vi "TabConAlt v0.2.vi"() -> ()   [LabVIEW 2017]
uses:
  <vilib>/Platform/TimedLoop/XDataNode/timing_clust.ctl
  <vilib>/Platform/TimedLoop/XDataNode/nitl_modes.ctl
  <vilib>/Platform/TimedLoop/XDataNode/wakeup.ctl
  <vilib>/Platform/TimedLoop/scheduler/LVUserAPI/_suppVIs/Create_1kHz_TSource.vi
  <vilib>/platform/TimedLoop/XDataNode/XDataNode.xnode
  <vilib>/ErrorRing/Error Ring.xnode
  <instrlib>/Stanford Research SR865/Stanford Research SR865.lvlib
  support/LIAinteraction/LIAinteraction.lvlib
  <vilib>/Platform/TimedLoop/XDataNode/XDNodeRunTimeDep.lvlib
panel:
  out "strMAT":string="Disconnected"
  in  "initMAT":bool
  out "statusMAT":bool
  out "connMAT":bool caption="Matisse TX"
  out "strMIL":string="Disconnected"
  in  "initMIL":bool
  out "statusMIL":bool
  out "connMIL":bool caption="Millenia eV 25W"
  out "strCCD":string="Disconnected"
  in  "initCCD":bool
  out "statusCCD":bool
  out "connCCD":bool caption="Pylon CCD"
  out "strSPT":string="Disconnected"
  in  "initSPT":bool caption="Spectrometer"
  out "statusSPT":bool
  out "connSPT":bool caption="Spectrometer"
  out "strLIA":string="Disconnected"
  in  "initLIA":bool caption="Lock-in"
  out "statusLIA":bool
  out "connLIA":bool caption="Lock-in & Chopper"
  in  "initALL":bool caption="Initialize all"
  in  "stopExecution":bool
  in  "clearNotifications":bool
  out "Notifications":string="\r\r\n"
  out "measRUN":bool caption="Measurement running"
  out "measREADY":bool caption="Measurement ready"
  out "UIbusy":bool caption="Interface busy"
  in  "Settings":T1(tab)=enum."Interface"
  in  "visaSPT":string caption="VISA address"
  in  "visaCCD":string caption="VISA address"
  out "unitChopFreq":string="Hz"
  in  "Linear ramp":dbl[unit]=200.0 min=1.0 max=500.0 step=1.0 format="%#_4g"
  in  "Start chopping":bool
  in  "findPrime":bool
  in  "visaLIA":string="visa://10.132.193.16/GPIB0::28::INSTR" caption="VISA address"
  in  "Chopping Frequency":dbl(knob)=1037.3807522912232 min=200.0 max=2000.0 step=1.0 scale=200.0..2000.0
  out "unitLinearRamp":string="Hz/s"
  in  "Ring cavity  energy":cluster{dbl[unit], dbl[unit]}(slide) caption="Ring cavity  energy / eV"
  in  "Ring cavity wavelength":cluster{dbl[unit], dbl[unit]}(slide)={0.0, 9.616279069767442e-07} caption="Ring cavity wavelength / nm"
  in  "Enslave Millennia eV":bool
  in  "Installed Optics":string(combo)="MOS2 BB"
  in  "visaMAT":string caption="VISA address"
  in  "Matisse Power":dbl[unit](knob)=1e-06 caption="Millenia Power" min=1.0 max=25.0 scale=1.0..25.0
  in  "visaMIL":string caption="VISA address"
  in  "Millenia Power":dbl[unit](knob)=0.001 min=1.0 max=25.0 scale=1.0..25.0
  in  "Hidden indicators":enum32{"General", "Sync"}(tab)
  out "LIAtimer1":bool
  out "TestInd2":bool
  out "MeasNum":dbl
  out "instrNum":dbl
  in  "actDummy":bool=TRUE
  out "DummyVisaOut":string
  in  "mainqSize":dbl=1000.0 caption="Queue size" min=1.0 step=1.0
  in  "timebaseMaster":dbl[unit]=0.08 caption="Master timebase" min=0.0001 max=0.5 step=0.0001 format="%#_6f"
  in  "timebaseSlave":dbl[unit]=0.16 caption="Slave timebase" min=0.0001 max=0.5 step=0.0001
  in  "abbrSPT":string="SPT"
  in  "abbrCCD":string="CCD"
  in  "abbrMIL":string="MIL"
  in  "abbrMAT":string="MAT"
  in  "abbrLIA":string="LIA"
  in  "nameSPT":string="Spectrometer"
  in  "nameLIA":string="SRS865"
  in  "nameCCD":string="Pylon CCD"
  in  "nameMIL":string="Millennia eV 25W"
  in  "nameMAT":string="Matisse 2 TX"
  # "Lower"
  # "Upper"
  # "eV"
  # "eV"
  # "Lower"
  # "Upper"
  # "nm"
  # "nm"
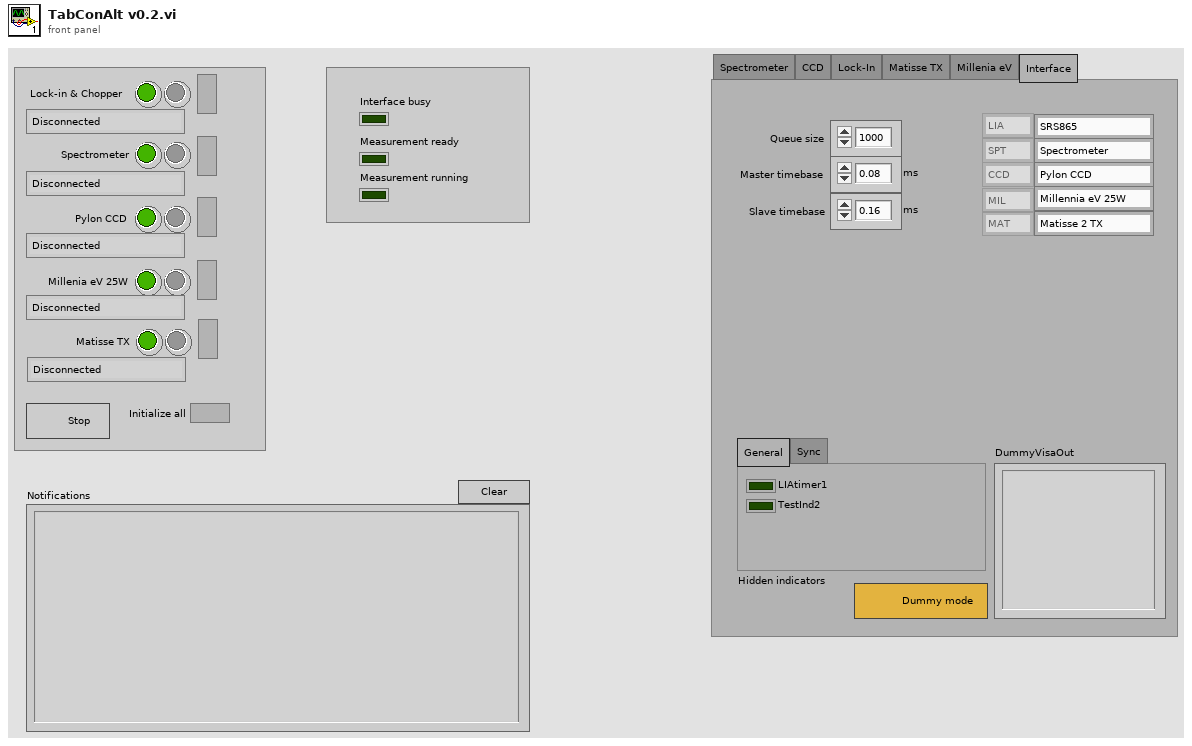
[diagram p1: front panel]
types:
  T1 = enum32{"Spectrometer", "CCD", "Lock-In", "Matisse TX", "Millenia eV", "Interface"}
  T2 = cluster{"elementArr":cluster{"cmd":string, "cmdclass":string, "data":variant}[]}
  T3 = cluster{"str":string, "ctlref":refnum<vi>, "newStatus":bool, "ctlstr":refnum<vi>}
  T4 = cluster{string, "chgStatusLED":refnum<user-event>}
  T5 = cluster{cluster{string, "chgStatusLED":refnum<user-event>}, cluster{string, "qintoMain":refnum<user-event>}}
  T6 = typedef "XDNodeRunTimeDep.lvlib/timing_clust.ctl" = cluster{"Expected End [f-1]":u64, "Actual End [f-1]":u64, "Finished Late? [f-1]":bool, "Expected End [i-1]":u64, "Actual End [i-1]":u64, "Finished Late? [i-1]":bool, "Expected Start [i]":u64, "Actual Start [i]":u64, "Expected Start [f]":u64, "Actual Start [f]":u64, "Source Name":string, "Structure Name":string, "Period":i64, "Deadline":i64, "Offset":i64, "Start":i64, "Priority":i32, "Timeout":i32, "Mode":T7, "Wakeup Reason":T8, "Error":errorcluster, "Source Type":string, "Secondary Source Type":string, "Global End Time":u64, "Global Start Time":u64, "Frame Duration":u64, "Iteration Duration":u64, "Assigned CPU":i32, "I/O Scan Engine Mode":u32}
  T7 = typedef "XDNodeRunTimeDep.lvlib/nitl_modes.ctl" = enum32{"No Change", "Process missed periods, maintain original phase", "Discard missed periods, maintain original phase", "Process missed periods, ignore original phase", "Discard missed periods, ignore original phase"}
  T8 = typedef "XDNodeRunTimeDep.lvlib/wakeup.ctl" = enum32{"Normal", "Aborted", "Asynchronous wakeup", "Timing source error", "Timed loop error", "Timeout"}
  T9 = typedef "RefArray.ctl" = cluster{"String":string, "Array":refnum<vi>[]}[]
  T10 = cluster{"Command":string, "Command class":string, "Variant":variant}
  T11 = cluster{"Command":string, "Command class":string, "Variant":variant}[]
  T12 = cluster{"cmd":string, "cmdclass":string, "data":variant}[]
  T13 = typedef "eventsource.ctl" = u32
  T14 = cluster{string, "abbrMAT":string, "Variant":variant}
  T15 = cluster{string, "abbrMAT":string, "Variant":variant}[]
  T16 = cluster{"String":string, "String 2":string, "Variant":variant}[]
  T17 = cluster{"String":string, "_chgStatusLED":refnum<user-event>}
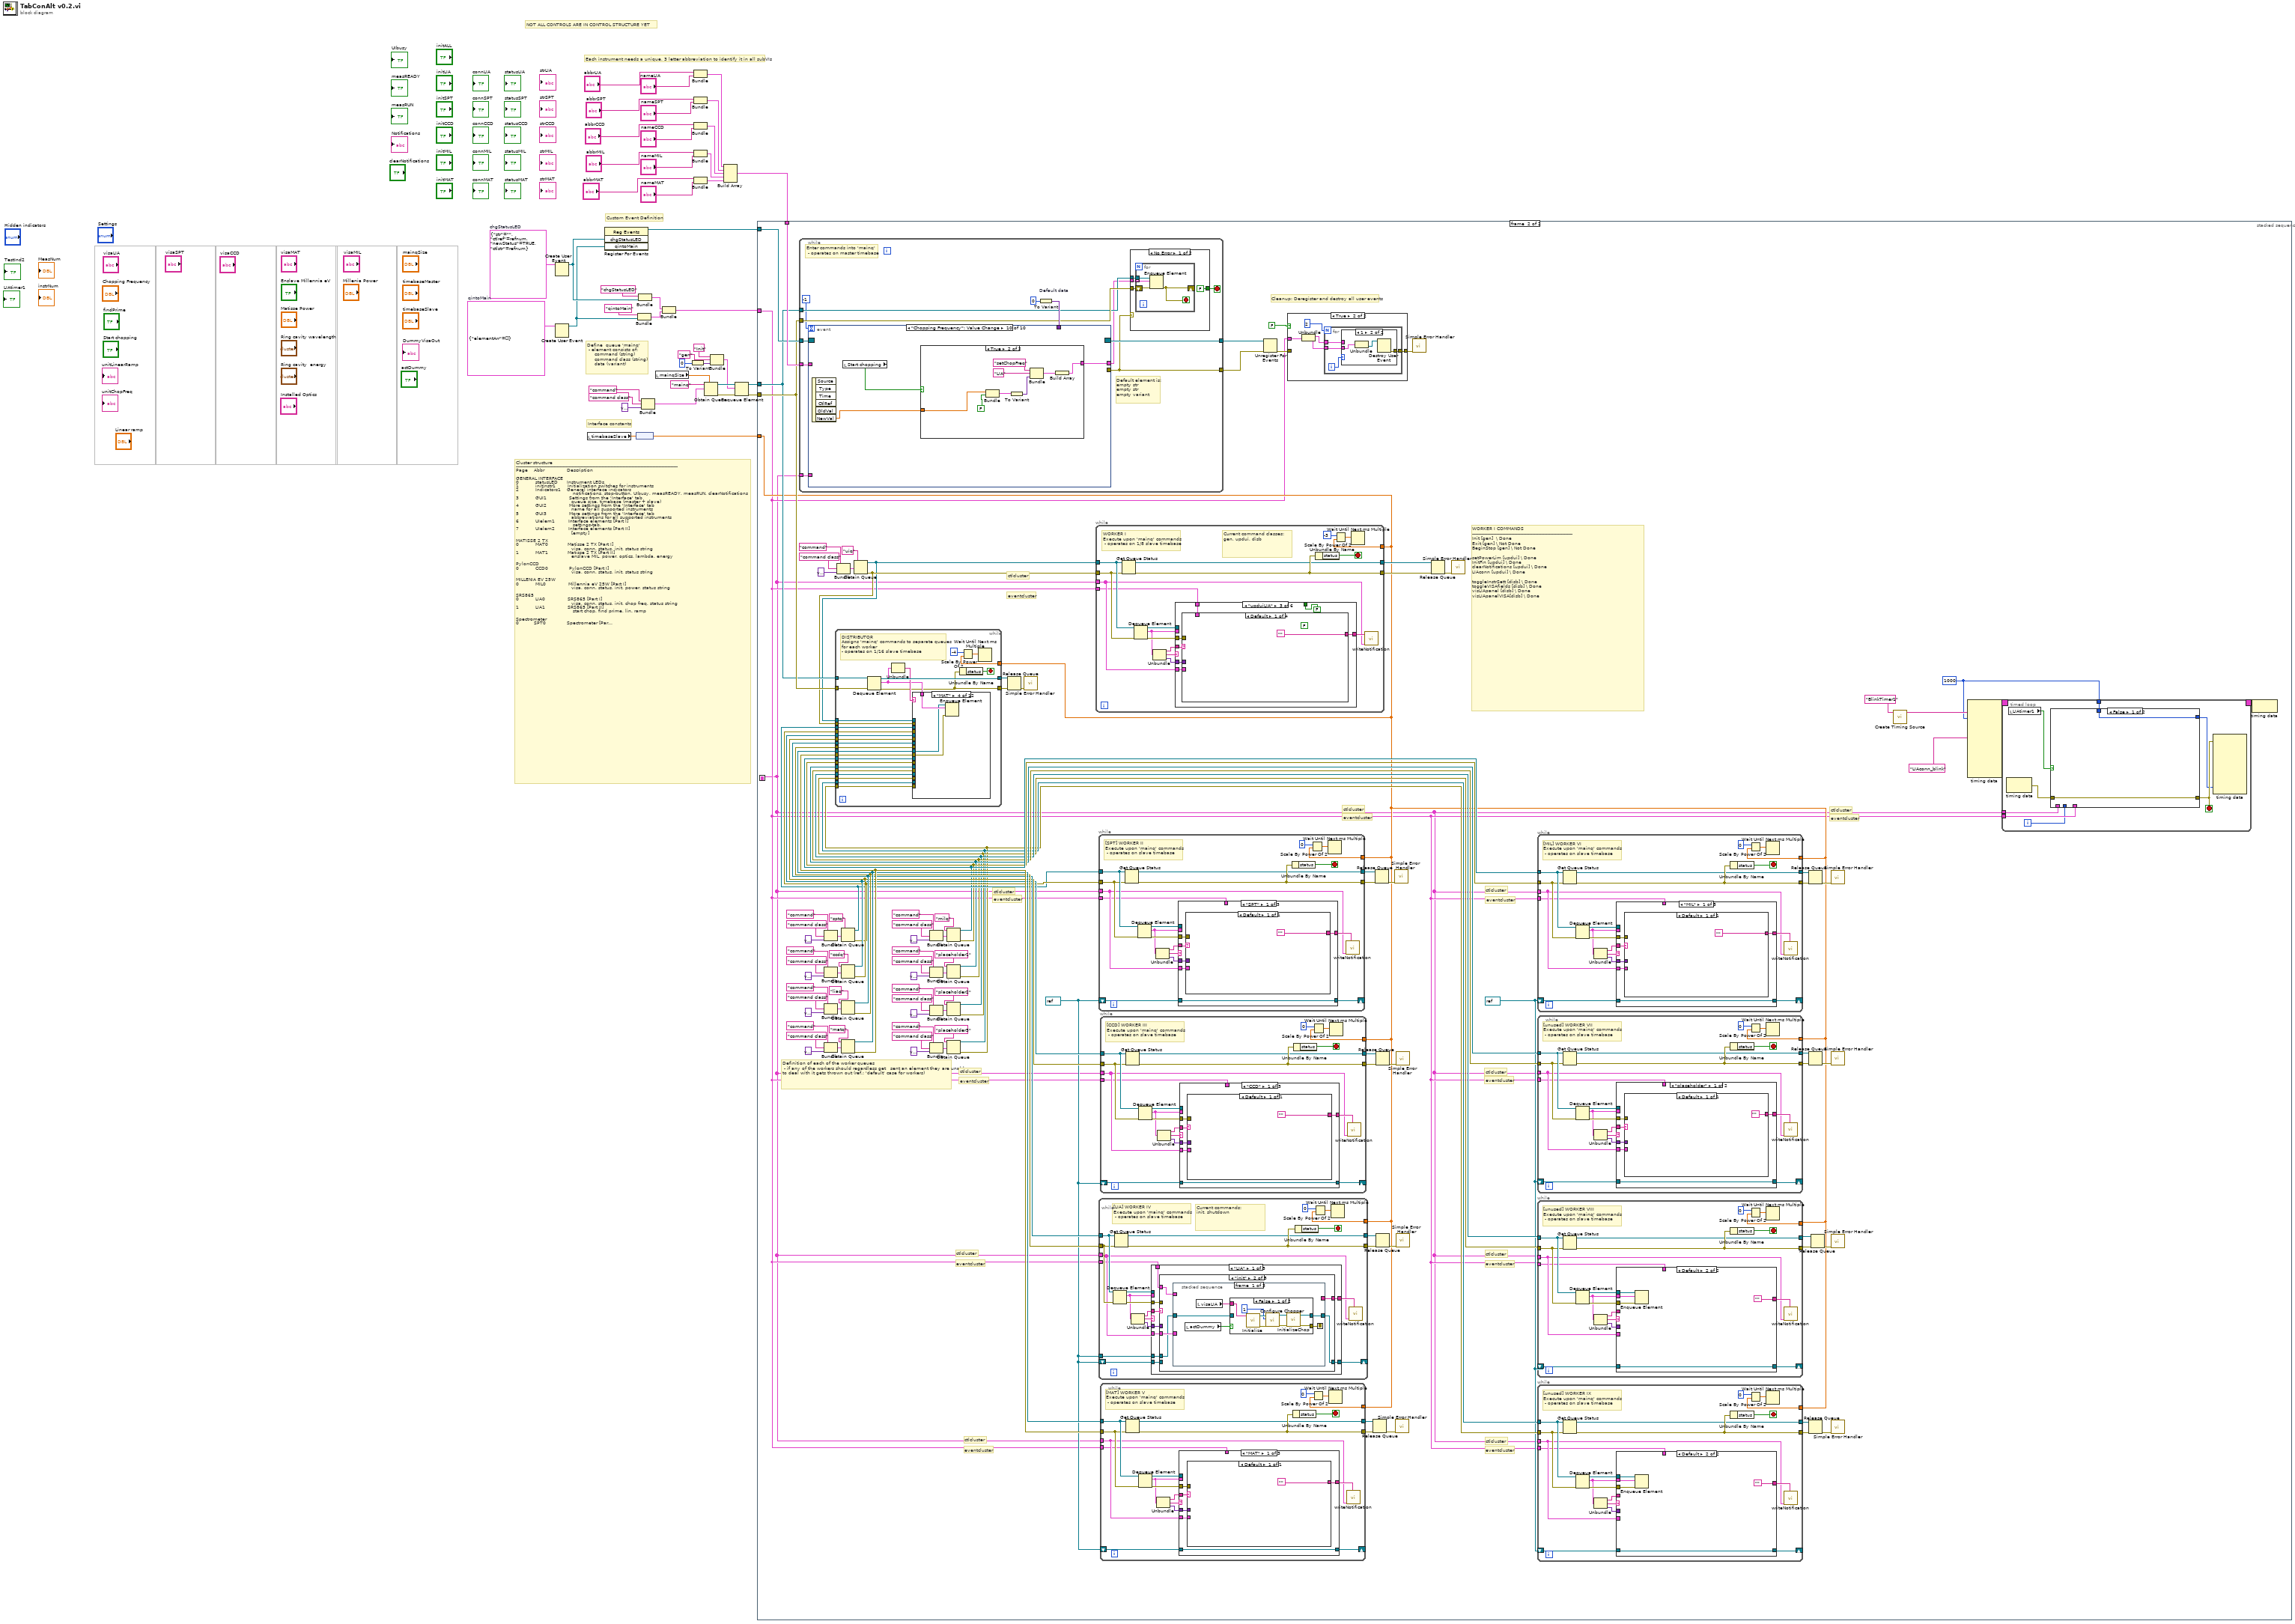
[diagram p0: block diagram]
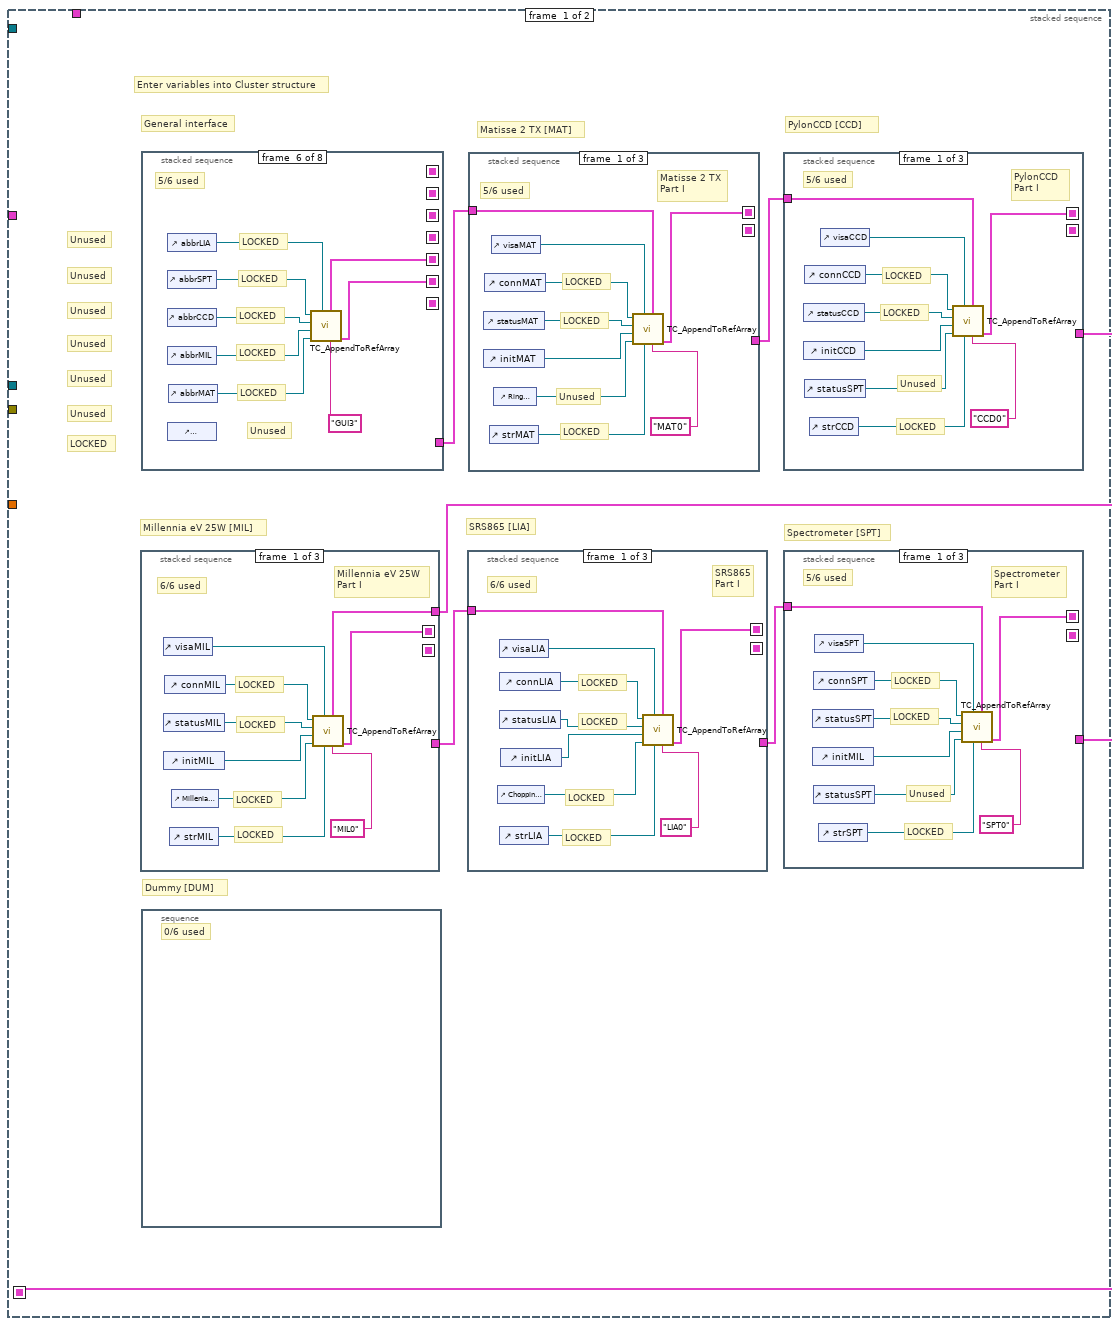
[diagram p2: hidden frame]
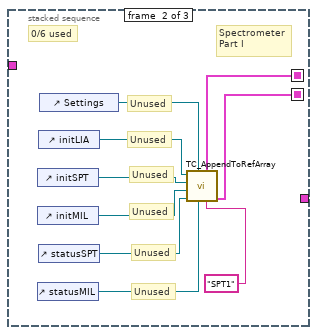
[diagram p3: hidden frame]
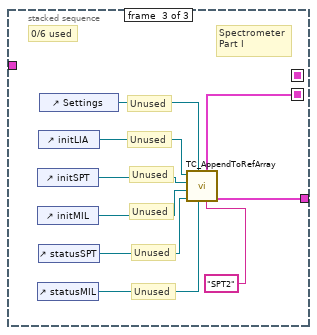
[diagram p4: hidden frame]
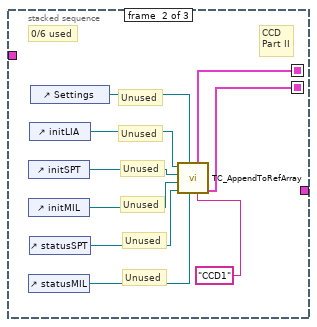
[diagram p5: hidden frame]
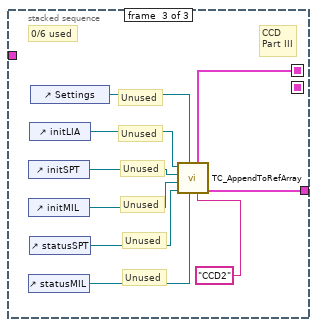
[diagram p6: hidden frame]
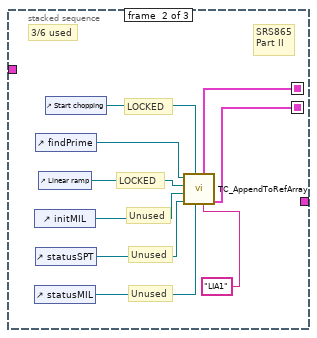
[diagram p7: hidden frame]
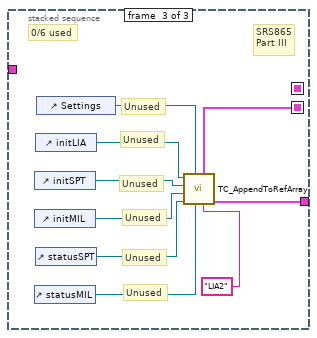
[diagram p8: hidden frame]
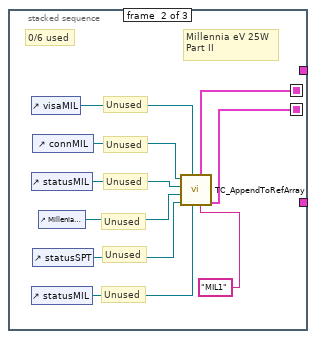
[diagram p9: hidden frame]
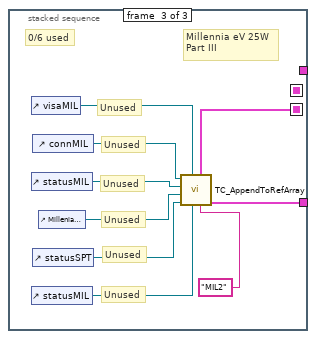
[diagram p10: hidden frame]
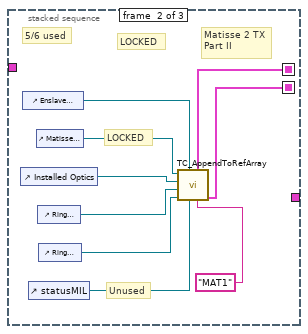
[diagram p11: hidden frame]
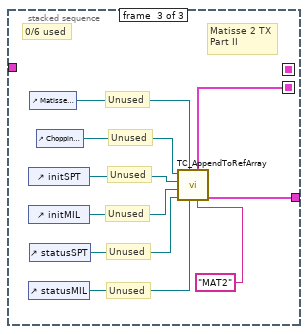
[diagram p12: hidden frame]
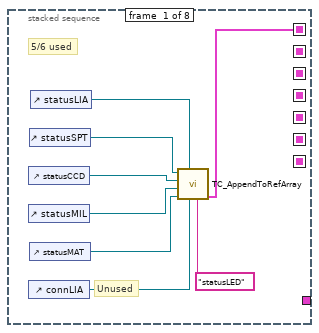
[diagram p13: hidden frame]
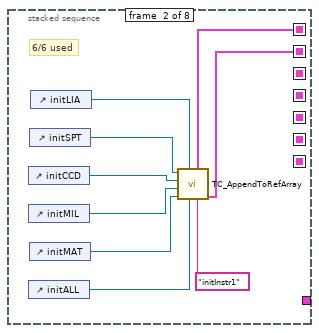
[diagram p14: hidden frame]
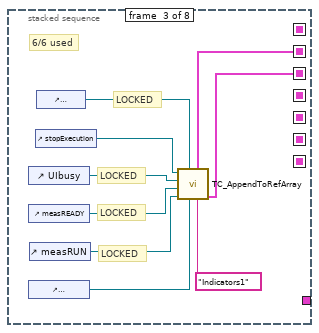
[diagram p15: hidden frame]
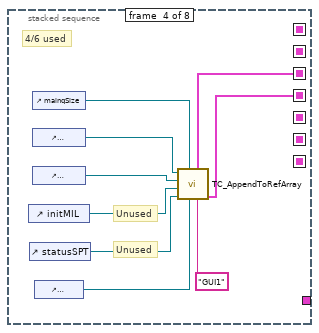
[diagram p16: hidden frame]
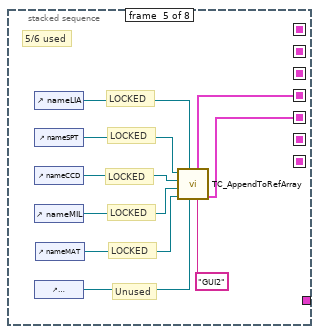
[diagram p17: hidden frame]
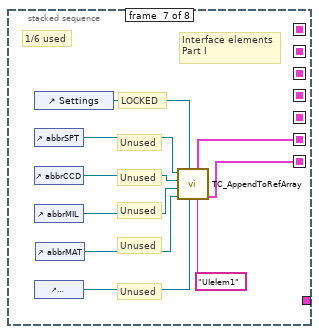
[diagram p18: hidden frame]
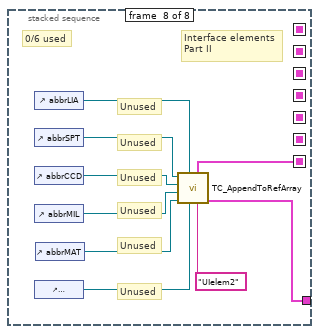
[diagram p19: hidden frame]
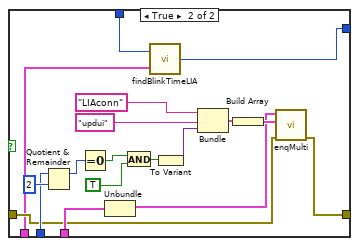
[diagram p20: hidden frame]
diagram:
  w13 = T2 {"elementArr"=[]}  # qintoMain
  w14 = T3 {"str"="", "ctlref"=refnum, "newStatus"=TRUE, "ctlstr"=refnum}  # chgStatusLED
  # "Custom Event Definition"
  # "Cluster structure\n------------------------------------------------------------------------------------------------------------\nPage    Abbr               Description\n\nGENERAL INTERFACE\n0           statusLED      Instrument LEDs\n1           initInstr1        Initialization switches for instruments\n2           Indicators1    General interface indicators\n                                      notifications, stop-button, UIbusy, measREADY, measRUN, clearNotifications\n3           GUI1               Settings from the 'Interface' tab\n                                     queue size, timebase (master + slave)\n4           GUI2               More settings from the 'Interface' tab\n                                     name for all supported instruments\n5           GUI3               More settings from the 'Interface' tab\n                                     abbreviations for all supported instruments\n6           UIelem1         Interface elements [Part I]\n                                      settings-tab,\n7           UIelem2         Interface elements [Part II]\n                                     [empty]\n\nMATISSE 2 TX\n0           MAT0             Matisse 2 TX [Part I]\n                                     visa, conn, status, init, status string\n1           MAT1             Matisse 2 TX [Part II]\n                                     enslave MIL, power, optics, lambda, energy\n\nPylonCCD\n0           CCD0              PylonCCD [Part I]\n                                     visa, conn, status, init, status string\n\nMILLENIA EV 25W\n0           MIL0               Millennia eV 25W [Part I]\n                                     visa, conn, status, init, power, status string\n\nSRS865\n0           LIA0               SRS865 [Part I]\n                                     visa, conn, status, init, chop freq, status string\n1           LIA1               SRS865 [Part II]\n                                      start chop, find prime, lin. ramp\n\nSpectrometer\n0          SPT0              Spectrometer [Part I]\n                                    visa, conn, status, init , status string"
  # "NOT ALL CONTROLS ARE IN CONTROL STRUCTURE YET"
  # "Each instrument needs a unique, 3 letter abbreviation to identify it in all subVIs"
  # "Define  queue 'mainq'\n - element consists of:\n     command (string)\n     command class (string)\n     data (variant)"
  # "Interface constants"
  n1 = Create User Event(user event datatype=w14) -> (user event=w12:refnum<user-event>)  [unwired: 1 in, 1 out]
  n2 = Create User Event(user event datatype=w13) -> (user event=w9:refnum<user-event>)  [unwired: 1 in, 1 out]
  n3 = local read "timebaseSlave"() -> (w33:dbl[unit])
  n4 = register-events(w12, w9) -> (reference out=w15:refnum<event-registration>)  [unwired: 2 in, 1 out]
  n5 = node(w33) -> (w32:dbl)
  n6 = Bundle("qintoMain", "qintoMain"=w9) -> (w2:cluster{string, "qintoMain":refnum<user-event>})  [unwired: 1 in]
  n7 = Bundle("chgStatusLED", "chgStatusLED"=w12) -> (w3:T4)  [unwired: 1 in]
  n8 = Bundle("command", "command class", variant) -> (w34:cluster{string, string, variant})  [unwired: 1 in]
  n9 = local read "mainqSize"() -> (w40:dbl)
  n10 = Bundle(w3, w2) -> (w1:T5)  [unwired: 1 in]
  n11 = To Variant(anything=0) -> (Variant=w42:variant)
  n12 = Bundle("abbrLIA"="abbrLIA", "nameLIA"="nameLIA") -> (w17:cluster{"abbrLIA":string, "nameLIA":string})  [unwired: 1 in]
  n13 = Bundle("abbrSPT"="abbrSPT", "nameSPT"="nameSPT") -> (w18:cluster{"abbrSPT":string, "nameSPT":string})  [unwired: 1 in]
  n14 = Bundle("abbrCCD"="abbrCCD", "nameCCD"="nameCCD") -> (w19:cluster{"abbrCCD":string, "nameCCD":string})  [unwired: 1 in]
  n15 = Bundle("abbrMIL"="abbrMIL", "nameMIL"="nameMIL") -> (w20:cluster{"abbrMIL":string, "nameMIL":string})  [unwired: 1 in]
  n16 = Bundle("abbrMAT"="abbrMAT", "nameMAT"="nameMAT") -> (w21:cluster{"abbrMAT":string, "nameMAT":string})  [unwired: 1 in]
  n17 = Obtain Queue(max queue size (-1, unlimited)=w40, name (unnamed)="mainq", element data type=w34) -> (queue out=w5:refnum<queue>, error out=w6:errorcluster)  [unwired: 2 in, 1 out]
  n18 = Bundle("Init", "gen", "Variant"=w42) -> (w4:cluster{string, string, "Variant":variant})  [unwired: 1 in]
  n19 = Build Array(w17, w18, w19, w20, w21) -> (w16:cluster{"abbrMAT":string, "nameMAT":string}[])
  n20 = Enqueue Element(queue=w5, element=w4, error in (no error)=w6) -> (queue out=w8:refnum<queue>, error out=w7:errorcluster)  [unwired: 1 in, 1 out]
  n21 = stacked-sequence {
    seq-local: [w44 _] -> [_ w258]
    tunnel: w32 -> [_ w262]
    tunnel: w16 -> [_ w359]
    tunnel: w15 -> [_ w355]
    tunnel: w1 -> [_ w259]
    tunnel: w8 -> [_ w350]
    tunnel: w7 -> [_ w351]
    frame #0 {
      # "LOCKED"
      # "Dummy [DUM]"
      # "Spectrometer [SPT]"
      # "PylonCCD [CCD]"
      # "Unused"
      # "Unused"
      # "Unused"
      # "Unused"
      # "Unused"
      # "Unused"
      # "SRS865 [LIA]"
      # "Millennia eV 25W [MIL]"
      # "General interface"
      # "Matisse 2 TX [MAT]"
      # "Enter variables into Cluster structure"
      n22 = stacked-sequence {
        seq-local: [w185 _ _ _ _ _ _ _] -> [_ w193 _ _ _ _ _ _]
        seq-local: [_ w194 _ _ _ _ _ _] -> [_ _ w204 _ _ _ _ _]
        seq-local: [_ _ w203 _ _ _ _ _] -> [_ _ _ w212 _ _ _ _]
        seq-local: [_ _ _ w211 _ _ _ _] -> [_ _ _ _ w221 _ _ _]
        seq-local: [_ _ _ _ w220 _ _ _] -> [_ _ _ _ _ w230 _ _]
        seq-local: [_ _ _ _ _ w229 _ _] -> [_ _ _ _ _ _ w238 _]
        seq-local: [_ _ _ _ _ _ w237 _] -> [_ _ _ _ _ _ _ w247]
        tunnel: [_ _ _ _ _ _ _ w246] -> w45
        frame #0 {
          # "Unused"
          # "5/6 used"
          n23 = control-ref of="statusCCD"() -> (w190:refnum<vi>)
          n24 = control-ref of="statusMIL"() -> (w189:refnum<vi>)
          n25 = control-ref of="connLIA"() -> (w187:refnum<vi>)
          n26 = control-ref of="statusSPT"() -> (w191:refnum<vi>)
          n27 = control-ref of="statusMAT"() -> (w188:refnum<vi>)
          n28 = control-ref of="statusLIA"() -> (w192:refnum<vi>)
          n29 = call "TC_AppendToRefArray.vi"("name"="statusLED", "ref6"=w187, "ref1"=w192, "ref5"=w188, "ref4"=w189, "ref3"=w190, "ref2"=w191) -> ("arrayOut"=w185:T9)  [unwired: 4 in]
        }
        frame #1 {
          # "6/6 used"
          n30 = control-ref of="initCCD"() -> (w199:refnum<vi>)
          n31 = control-ref of="initMIL"() -> (w198:refnum<vi>)
          n32 = control-ref of="initALL"() -> (w196:refnum<vi>)
          n33 = control-ref of="initSPT"() -> (w200:refnum<vi>)
          n34 = control-ref of="initMAT"() -> (w197:refnum<vi>)
          n35 = control-ref of="initLIA"() -> (w201:refnum<vi>)
          n36 = call "TC_AppendToRefArray.vi"("name"="initInstr1", "arrayIn"=w193, "ref6"=w196, "ref1"=w201, "ref5"=w197, "ref4"=w198, "ref3"=w199, "ref2"=w200) -> ("arrayOut"=w194:T9)  [unwired: 3 in]
        }
        frame #2 {
          # "LOCKED"
          # "LOCKED"
          # "LOCKED"
          # "LOCKED"
          # "6/6 used"
          n37 = control-ref of="UIbusy"() -> (w209:refnum<vi>)
          n38 = control-ref of="measREADY"() -> (w208:refnum<vi>)
          n39 = control-ref of="clearNotifications"() -> (w206:refnum<vi>)
          n40 = control-ref of="measRUN"() -> (w207:refnum<vi>)
          n41 = control-ref of="stopExecution"() -> (w202:refnum<vi>)
          n42 = control-ref of="Notifications"() -> (w210:refnum<vi>)
          n43 = call "TC_AppendToRefArray.vi"("name"="Indicators1", "arrayIn"=w204, "ref6"=w206, "ref1"=w210, "ref5"=w207, "ref4"=w208, "ref3"=w209, "ref2"=w202) -> ("arrayOut"=w203:T9)  [unwired: 3 in]
        }
        frame #3 {
          # "Unused"
          # "Unused"
          # "4/6 used"
          n44 = control-ref of="initMIL"() -> (w216:refnum<vi>)
          n45 = control-ref of="statusSPT"() -> (w215:refnum<vi>)
          n46 = control-ref of="mainqSize"() -> (w219:refnum<vi>)
          n47 = control-ref of="timebaseMaster"() -> (w218:refnum<vi>)
          n48 = control-ref of="timebaseSlave"() -> (w217:refnum<vi>)
          n49 = control-ref of="DummyVisaOut"() -> (w214:refnum<vi>)
          n50 = call "TC_AppendToRefArray.vi"("name"="GUI1", "arrayIn"=w212, "ref6"=w214, "ref1"=w219, "ref5"=w215, "ref4"=w216, "ref3"=w217, "ref2"=w218) -> ("arrayOut"=w211:T9)  [unwired: 3 in]
        }
        frame #4 {
          # "LOCKED"
          # "LOCKED"
          # "LOCKED"
          # "LOCKED"
          # "LOCKED"
          # "Unused"
          # "5/6 used"
          n51 = control-ref of="nameLIA"() -> (w228:refnum<vi>)
          n52 = control-ref of="nameSPT"() -> (w227:refnum<vi>)
          n53 = control-ref of="nameCCD"() -> (w226:refnum<vi>)
          n54 = control-ref of="nameMIL"() -> (w225:refnum<vi>)
          n55 = control-ref of="DummyVisaOut"() -> (w223:refnum<vi>)
          n56 = control-ref of="nameMAT"() -> (w224:refnum<vi>)
          n57 = call "TC_AppendToRefArray.vi"("name"="GUI2", "arrayIn"=w221, "ref6"=w223, "ref1"=w228, "ref5"=w224, "ref4"=w225, "ref3"=w226, "ref2"=w227) -> ("arrayOut"=w220:T9)  [unwired: 3 in]
        }
        frame #5 {
          # "LOCKED"
          # "LOCKED"
          # "LOCKED"
          # "LOCKED"
          # "LOCKED"
          # "Unused"
          # "5/6 used"
          n58 = control-ref of="abbrLIA"() -> (w236:refnum<vi>)
          n59 = control-ref of="abbrSPT"() -> (w235:refnum<vi>)
          n60 = control-ref of="abbrCCD"() -> (w234:refnum<vi>)
          n61 = control-ref of="abbrMIL"() -> (w233:refnum<vi>)
          n62 = control-ref of="DummyVisaOut"() -> ()  [unwired: 1 out]
          n63 = control-ref of="abbrMAT"() -> (w232:refnum<vi>)
          n64 = call "TC_AppendToRefArray.vi"("name"="GUI3", "arrayIn"=w230, "ref1"=w236, "ref5"=w232, "ref4"=w233, "ref3"=w234, "ref2"=w235) -> ("arrayOut"=w229:T9)  [unwired: 4 in]
        }
        frame #6 {
          # "LOCKED"
          # "Interface elements\nPart I"
          # "Unused"
          # "Unused"
          # "Unused"
          # "Unused"
          # "Unused"
          # "1/6 used"
          n65 = control-ref of="Settings"() -> (w245:refnum<vi>)
          n66 = control-ref of="abbrSPT"() -> (w244:refnum<vi>)
          n67 = control-ref of="abbrCCD"() -> (w243:refnum<vi>)
          n68 = control-ref of="abbrMIL"() -> (w242:refnum<vi>)
          n69 = control-ref of="DummyVisaOut"() -> (w240:refnum<vi>)
          n70 = control-ref of="abbrMAT"() -> (w241:refnum<vi>)
          n71 = call "TC_AppendToRefArray.vi"("name"="UIelem1", "arrayIn"=w238, "ref6"=w240, "ref1"=w245, "ref5"=w241, "ref4"=w242, "ref3"=w243, "ref2"=w244) -> ("arrayOut"=w237:T9)  [unwired: 3 in]
        }
        frame #7 {
          # "Interface elements\nPart II"
          # "Unused"
          # "Unused"
          # "Unused"
          # "Unused"
          # "Unused"
          # "Unused"
          # "0/6 used"
          n72 = control-ref of="abbrLIA"() -> (w254:refnum<vi>)
          n73 = control-ref of="abbrSPT"() -> (w253:refnum<vi>)
          n74 = control-ref of="abbrCCD"() -> (w252:refnum<vi>)
          n75 = control-ref of="abbrMIL"() -> (w251:refnum<vi>)
          n76 = control-ref of="DummyVisaOut"() -> (w249:refnum<vi>)
          n77 = control-ref of="abbrMAT"() -> (w250:refnum<vi>)
          n78 = call "TC_AppendToRefArray.vi"("name"="UIelem2", "arrayIn"=w247, "ref6"=w249, "ref1"=w254, "ref5"=w250, "ref4"=w251, "ref3"=w252, "ref2"=w253) -> ("arrayOut"=w246:T9)  [unwired: 3 in]
        }
      }
      n79 = stacked-sequence {
        frame #0 {
          # "0/6 used"
        }
      }
      n80 = stacked-sequence {
        seq-local: [w158 _ _] -> [_ w168 _]
        seq-local: [_ w167 _] -> [_ _ w176]
        tunnel: w45 -> [w159 _ _]
        tunnel: [_ _ w177] -> w47
        frame #0 {
          # "LOCKED"
          # "LOCKED"
          # "LOCKED"
          # "Unused"
          # "Matisse 2 TX\nPart I"
          # "5/6 used"
          n81 = control-ref of="statusMAT"() -> (w163:refnum<vi>)
          n82 = control-ref of="initMAT"() -> (w164:refnum<vi>)
          n83 = control-ref of="connMAT"() -> (w162:refnum<vi>)
          n84 = control-ref of="strMAT"() -> (w166:refnum<vi>)
          n85 = control-ref of="visaMAT"() -> (w161:refnum<vi>)
          n86 = control-ref of="Ring cavity  energy"() -> (w165:refnum<vi>)
          n87 = call "TC_AppendToRefArray.vi"("name"="MAT0", "arrayIn"=w159, "ref6"=w166, "ref1"=w161, "ref5"=w165, "ref4"=w164, "ref3"=w163, "ref2"=w162) -> ("arrayOut"=w158:T9)  [unwired: 3 in]
        }
        frame #1 {
          # "LOCKED"
          # "LOCKED"
          # "Unused"
          # "Matisse 2 TX\nPart II"
          # "5/6 used"
          n88 = control-ref of="Installed Optics"() -> (w172:refnum<vi>)
          n89 = control-ref of="Enslave Millennia eV"() -> (w170:refnum<vi>)
          n90 = control-ref of="statusMIL"() -> (w175:refnum<vi>)
          n91 = control-ref of="Matisse Power"() -> (w171:refnum<vi>)
          n92 = control-ref of="Ring cavity wavelength"() -> (w173:refnum<vi>)
          n93 = control-ref of="Ring cavity  energy"() -> (w174:refnum<vi>)
          n94 = call "TC_AppendToRefArray.vi"("name"="MAT1", "arrayIn"=w168, "ref6"=w175, "ref1"=w170, "ref5"=w174, "ref4"=w173, "ref3"=w172, "ref2"=w171) -> ("arrayOut"=w167:T9)  [unwired: 3 in]
        }
        frame #2 {
          # "Unused"
          # "Unused"
          # "Unused"
          # "Unused"
          # "Unused"
          # "Unused"
          # "Matisse 2 TX\nPart II"
          # "0/6 used"
          n95 = control-ref of="initSPT"() -> (w181:refnum<vi>)
          n96 = control-ref of="initMIL"() -> (w182:refnum<vi>)
          n97 = control-ref of="statusMIL"() -> (w184:refnum<vi>)
          n98 = control-ref of="Matisse Power"() -> (w179:refnum<vi>)
          n99 = control-ref of="statusSPT"() -> (w183:refnum<vi>)
          n100 = control-ref of="Chopping Frequency"() -> (w180:refnum<vi>)
          n101 = call "TC_AppendToRefArray.vi"("name"="MAT2", "arrayIn"=w176, "ref6"=w184, "ref1"=w179, "ref5"=w183, "ref4"=w182, "ref3"=w181, "ref2"=w180) -> ("arrayOut"=w177:T9)  [unwired: 3 in]
        }
      }
      n102 = stacked-sequence {
        seq-local: [w77 _ _] -> [_ w87 w96]
        seq-local: [_ w86 _] -> [_ _ _]
        tunnel: w47 -> [w78 _ _]
        tunnel: [_ _ w95] -> w48
        frame #0 {
          # "LOCKED"
          # "LOCKED"
          # "LOCKED"
          # "PylonCCD\nPart I"
          # "Unused"
          # "5/6 used"
          n103 = control-ref of="statusCCD"() -> (w82:refnum<vi>)
          n104 = control-ref of="initCCD"() -> (w83:refnum<vi>)
          n105 = control-ref of="connCCD"() -> (w81:refnum<vi>)
          n106 = control-ref of="statusSPT"() -> (w84:refnum<vi>)
          n107 = control-ref of="strCCD"() -> (w85:refnum<vi>)
          n108 = control-ref of="visaCCD"() -> (w80:refnum<vi>)
          n109 = call "TC_AppendToRefArray.vi"("name"="CCD0", "arrayIn"=w78, "ref6"=w85, "ref1"=w80, "ref5"=w84, "ref4"=w83, "ref3"=w82, "ref2"=w81) -> ("arrayOut"=w77:T9)  [unwired: 3 in]
        }
        frame #1 {
          # "CCD\nPart II"
          # "Unused"
          # "Unused"
          # "Unused"
          # "Unused"
          # "Unused"
          # "Unused"
          # "0/6 used"
          n110 = control-ref of="initSPT"() -> (w91:refnum<vi>)
          n111 = control-ref of="initMIL"() -> (w92:refnum<vi>)
          n112 = control-ref of="statusMIL"() -> (w94:refnum<vi>)
          n113 = control-ref of="initLIA"() -> (w90:refnum<vi>)
          n114 = control-ref of="statusSPT"() -> (w93:refnum<vi>)
          n115 = control-ref of="Settings"() -> (w89:refnum<vi>)
          n116 = call "TC_AppendToRefArray.vi"("name"="CCD1", "arrayIn"=w87, "ref6"=w94, "ref1"=w89, "ref5"=w93, "ref4"=w92, "ref3"=w91, "ref2"=w90) -> ("arrayOut"=w86:T9)  [unwired: 3 in]
        }
        frame #2 {
          # "CCD\nPart III"
          # "Unused"
          # "Unused"
          # "Unused"
          # "Unused"
          # "Unused"
          # "Unused"
          # "0/6 used"
          n117 = control-ref of="initSPT"() -> (w100:refnum<vi>)
          n118 = control-ref of="initMIL"() -> (w101:refnum<vi>)
          n119 = control-ref of="statusMIL"() -> (w103:refnum<vi>)
          n120 = control-ref of="initLIA"() -> (w99:refnum<vi>)
          n121 = control-ref of="statusSPT"() -> (w102:refnum<vi>)
          n122 = control-ref of="Settings"() -> (w98:refnum<vi>)
          n123 = call "TC_AppendToRefArray.vi"("name"="CCD2", "arrayIn"=w96, "ref6"=w103, "ref1"=w98, "ref5"=w102, "ref4"=w101, "ref3"=w100, "ref2"=w99) -> ("arrayOut"=w95:T9)  [unwired: 3 in]
        }
      }
      n124 = stacked-sequence {
        seq-local: [w131 _ _] -> [_ w141 _]
        seq-local: [_ w140 _] -> [_ _ w150]
        tunnel: w48 -> [w132 _ _]
        tunnel: [_ _ w149] -> w46
        frame #0 {
          # "LOCKED"
          # "LOCKED"
          # "LOCKED"
          # "LOCKED"
          # "Millennia eV 25W\nPart I"
          # "6/6 used"
          n125 = control-ref of="visaMIL"() -> (w134:refnum<vi>)
          n126 = control-ref of="statusMIL"() -> (w136:refnum<vi>)
          n127 = control-ref of="initMIL"() -> (w137:refnum<vi>)
          n128 = control-ref of="connMIL"() -> (w135:refnum<vi>)
          n129 = control-ref of="strMIL"() -> (w139:refnum<vi>)
          n130 = control-ref of="Millenia Power"() -> (w138:refnum<vi>)
          n131 = call "TC_AppendToRefArray.vi"("name"="MIL0", "arrayIn"=w132, "ref6"=w139, "ref1"=w134, "ref5"=w138, "ref4"=w137, "ref3"=w136, "ref2"=w135) -> ("arrayOut"=w131:T9)  [unwired: 3 in]
        }
        frame #1 {
          # "Unused"
          # "Unused"
          # "Unused"
          # "Unused"
          # "Unused"
          # "Unused"
          # "Millennia eV 25W\nPart II"
          # "0/6 used"
          n132 = control-ref of="visaMIL"() -> (w143:refnum<vi>)
          n133 = control-ref of="statusMIL"() -> (w145:refnum<vi>)
          n134 = control-ref of="statusMIL"() -> (w148:refnum<vi>)
          n135 = control-ref of="connMIL"() -> (w144:refnum<vi>)
          n136 = control-ref of="statusSPT"() -> (w147:refnum<vi>)
          n137 = control-ref of="Millenia Power"() -> (w146:refnum<vi>)
          n138 = call "TC_AppendToRefArray.vi"("name"="MIL1", "arrayIn"=w141, "ref6"=w148, "ref1"=w143, "ref5"=w147, "ref4"=w146, "ref3"=w145, "ref2"=w144) -> ("arrayOut"=w140:T9)  [unwired: 3 in]
        }
        frame #2 {
          # "Unused"
          # "Unused"
          # "Unused"
          # "Unused"
          # "Unused"
          # "Unused"
          # "Millennia eV 25W\nPart III"
          # "0/6 used"
          n139 = control-ref of="visaMIL"() -> (w152:refnum<vi>)
          n140 = control-ref of="statusMIL"() -> (w154:refnum<vi>)
          n141 = control-ref of="statusMIL"() -> (w157:refnum<vi>)
          n142 = control-ref of="connMIL"() -> (w153:refnum<vi>)
          n143 = control-ref of="statusSPT"() -> (w156:refnum<vi>)
          n144 = control-ref of="Millenia Power"() -> (w155:refnum<vi>)
          n145 = call "TC_AppendToRefArray.vi"("name"="MIL2", "arrayIn"=w150, "ref6"=w157, "ref1"=w152, "ref5"=w156, "ref4"=w155, "ref3"=w154, "ref2"=w153) -> ("arrayOut"=w149:T9)  [unwired: 3 in]
        }
      }
      n146 = stacked-sequence {
        seq-local: [w108 _ _] -> [_ w114 _]
        seq-local: [_ w113 _] -> [_ _ w122]
        tunnel: w46 -> [w109 _ _]
        tunnel: [_ _ w123] -> w49
        frame #0 {
          # "LOCKED"
          # "LOCKED"
          # "LOCKED"
          # "LOCKED"
          # "SRS865\nPart I"
          # "6/6 used"
          n147 = control-ref of="Chopping Frequency"() -> (w107:refnum<vi>)
          n148 = control-ref of="visaLIA"() -> (w111:refnum<vi>)
          n149 = control-ref of="connLIA"() -> (w104:refnum<vi>)
          n150 = control-ref of="statusLIA"() -> (w105:refnum<vi>)
          n151 = control-ref of="strLIA"() -> (w112:refnum<vi>)
          n152 = control-ref of="initLIA"() -> (w106:refnum<vi>)
          n153 = call "TC_AppendToRefArray.vi"("name"="LIA0", "arrayIn"=w109, "ref6"=w112, "ref1"=w111, "ref5"=w107, "ref4"=w106, "ref3"=w105, "ref2"=w104) -> ("arrayOut"=w108:T9)  [unwired: 3 in]
        }
        frame #1 {
          # "LOCKED"
          # "LOCKED"
          # "Unused"
          # "Unused"
          # "Unused"
          # "SRS865\nPart II"
          # "3/6 used"
          n154 = control-ref of="initMIL"() -> (w119:refnum<vi>)
          n155 = control-ref of="statusMIL"() -> (w121:refnum<vi>)
          n156 = control-ref of="findPrime"() -> (w117:refnum<vi>)
          n157 = control-ref of="statusSPT"() -> (w120:refnum<vi>)
          n158 = control-ref of="Linear ramp"() -> (w118:refnum<vi>)
          n159 = control-ref of="Start chopping"() -> (w116:refnum<vi>)
          n160 = call "TC_AppendToRefArray.vi"("name"="LIA1", "arrayIn"=w114, "ref6"=w121, "ref1"=w116, "ref5"=w120, "ref4"=w119, "ref3"=w118, "ref2"=w117) -> ("arrayOut"=w113:T9)  [unwired: 3 in]
        }
        frame #2 {
          # "Unused"
          # "Unused"
          # "Unused"
          # "Unused"
          # "Unused"
          # "Unused"
          # "SRS865\nPart III"
          # "0/6 used"
          n161 = control-ref of="initSPT"() -> (w127:refnum<vi>)
          n162 = control-ref of="initMIL"() -> (w128:refnum<vi>)
          n163 = control-ref of="statusMIL"() -> (w130:refnum<vi>)
          n164 = control-ref of="initLIA"() -> (w126:refnum<vi>)
          n165 = control-ref of="statusSPT"() -> (w129:refnum<vi>)
          n166 = control-ref of="Settings"() -> (w125:refnum<vi>)
          n167 = call "TC_AppendToRefArray.vi"("name"="LIA2", "arrayIn"=w122, "ref6"=w130, "ref1"=w125, "ref5"=w129, "ref4"=w128, "ref3"=w127, "ref2"=w126) -> ("arrayOut"=w123:T9)  [unwired: 3 in]
        }
      }
      n168 = stacked-sequence {
        seq-local: [w50 _ _] -> [_ w60 _]
        seq-local: [_ w59 _] -> [_ _ w69]
        tunnel: w49 -> [w51 _ _]
        tunnel: [_ _ w68] -> w44
        frame #0 {
          # "LOCKED"
          # "LOCKED"
          # "LOCKED"
          # "Spectrometer\nPart I"
          # "Unused"
          # "5/6 used"
          n169 = control-ref of="statusSPT"() -> (w55:refnum<vi>)
          n170 = control-ref of="initMIL"() -> (w56:refnum<vi>)
          n171 = control-ref of="connSPT"() -> (w54:refnum<vi>)
          n172 = control-ref of="statusSPT"() -> (w57:refnum<vi>)
          n173 = control-ref of="visaSPT"() -> (w53:refnum<vi>)
          n174 = control-ref of="strSPT"() -> (w58:refnum<vi>)
          n175 = call "TC_AppendToRefArray.vi"("name"="SPT0", "arrayIn"=w51, "ref6"=w58, "ref1"=w53, "ref5"=w57, "ref4"=w56, "ref3"=w55, "ref2"=w54) -> ("arrayOut"=w50:T9)  [unwired: 3 in]
        }
        frame #1 {
          # "Spectrometer\nPart I"
          # "Unused"
          # "Unused"
          # "Unused"
          # "Unused"
          # "Unused"
          # "Unused"
          # "0/6 used"
          n176 = control-ref of="initSPT"() -> (w64:refnum<vi>)
          n177 = control-ref of="initMIL"() -> (w65:refnum<vi>)
          n178 = control-ref of="statusMIL"() -> (w67:refnum<vi>)
          n179 = control-ref of="initLIA"() -> (w63:refnum<vi>)
          n180 = control-ref of="statusSPT"() -> (w66:refnum<vi>)
          n181 = control-ref of="Settings"() -> (w62:refnum<vi>)
          n182 = call "TC_AppendToRefArray.vi"("name"="SPT1", "arrayIn"=w60, "ref6"=w67, "ref1"=w62, "ref5"=w66, "ref4"=w65, "ref3"=w64, "ref2"=w63) -> ("arrayOut"=w59:T9)  [unwired: 3 in]
        }
        frame #2 {
          # "Spectrometer\nPart I"
          # "Unused"
          # "Unused"
          # "Unused"
          # "Unused"
          # "Unused"
          # "Unused"
          # "0/6 used"
          n183 = control-ref of="initSPT"() -> (w73:refnum<vi>)
          n184 = control-ref of="initMIL"() -> (w74:refnum<vi>)
          n185 = control-ref of="statusMIL"() -> (w76:refnum<vi>)
          n186 = control-ref of="initLIA"() -> (w72:refnum<vi>)
          n187 = control-ref of="statusSPT"() -> (w75:refnum<vi>)
          n188 = control-ref of="Settings"() -> (w71:refnum<vi>)
          n189 = call "TC_AppendToRefArray.vi"("name"="SPT2", "arrayIn"=w69, "ref6"=w76, "ref1"=w71, "ref5"=w75, "ref4"=w74, "ref3"=w73, "ref2"=w72) -> ("arrayOut"=w68:T9)  [unwired: 3 in]
        }
      }
    }
    frame #1 {
      w255 = 1000
      w265 = refnum<visa-resource-name> refnum ("VISA resource name out")
      w264 = refnum<visa-resource-name> refnum ("VISA resource name out")
      # "ctlcluster"
      # "eventcluster"
      # "ctlcluster"
      # "eventcluster"
      # "ctlcluster"
      # "eventcluster"
      # "ctlcluster"
      # "eventcluster"
      # "ctlcluster"
      # "eventcluster"
      # "ctlcluster"
      # "eventcluster"
      # "ctlcluster"
      # "eventcluster"
      # "ctlcluster"
      # "eventcluster"
      # "Cleanup: Deregister and destroy all user events"
      # "ctlcluster"
      # "eventcluster"
      # "ctlcluster"
      # "eventcluster"
      # "ctlcluster"
      # "eventcluster"
      # "WORKER I COMMANDS\n-------------------------------------------------------------------\nInit [gen]  \\ Done\nExit [gen] \\ Not Done\nBeginStop [gen] \\ Not Done\n\nsetPowerLim [updui] \\ Done\nInitFin [updui] \\ Done\nclearNotifications [updui] \\ Done\nLIAconn [updui] \\ Done\n\ntoggleInstrSett [disb] \\ Done \ntoggleVISAfields [disb] \\ Done\nvisLIApanel [disb] \\ Done\nvisLIApanelVISA[disb] \\ Done"
      # "Definition of each of the worker queues\n - if any of the workers should regardless get   sent an element they are unable to deal with it gets thrown out (ref.: 'default' case for workers)"
      n190 = while {
        tunnel: w350 -> [w1116]
        tunnel: w351 -> [w1117]
        tunnel: w359 -> [w1113]
        tunnel: w258 -> [w1112]
        tunnel: [w1110] -> w356
        tunnel: w355 -> [w1119]
        tunnel: [w1118] -> w364
        stop <- w1115 stop-if-true
        # "Default element is:\nempty str\nempty str\nempty variant"
        # "Enter commands into 'mainq'\n - operates on master timebase"
        n191 = To Variant "Default data"(anything=0) -> (Variant=w1121:variant)
        n192 = event shown="[9] \"Chopping Frequency\": Value Change" {
          selector: w1119 -> [_ _ _ _ _ _ _ _ _ _]
          dyn-events: [_ _ _ _ _ _ _ _ _ _] -> w1118
          timeout: -1 -> [_ _ _ _ _ _ _ _ _ _]
          tunnel: w1121 -> [_ w1141 w1144 _ w1156 _ _ _ _ _]
          tunnel: [_ w1142 w1147 _ w1157 _ w1187 w1196 w1241 w1248] -> w1114
          tunnel: w1113 -> [_ _ _ _ _ _ _ w1208 _ _]
          tunnel: w1112 -> [_ _ _ _ _ _ _ w1198 _ _]
          tunnel: [_ _ _ _ _ w1166 _ _ _ _] -> w1110
          event Timeout {
            n193 = event-data() -> ()  [unwired: 1 in, 3 out]
          }
          event "stopExecution": Value Change {
            w1139 = "gen"  # Command class
            w1138 = "BeginStop"  # Command
            n194 = event-data() -> ()  [unwired: 1 in, 3 out]
            n195 = Bundle("Command"=w1138, "Command class"=w1139, "Variant"=w1141) -> (w1140:T10)  [unwired: 1 in]
            n196 = Build Array(w1140) -> (w1142:T11)
          }
          event Panel Close? {
            w1145 = "gen"  # Command class
            w1146 = "Exit"  # Command
            n197 = event-data() -> ()  [unwired: 1 in, 4 out]
            n198 = Bundle("Command"=w1146, "Command class"=w1145, "Variant"=w1144) -> (w1143:T10)  [unwired: 1 in]
            n199 = event-data() -> ()  [unwired: 2 in, 1 out]
            n200 = Build Array(w1143) -> (w1147:T11)
          }
          event User Event {
            n201 = event-data() -> ("str"=w1148:string, "ctlref"=w1151:refnum<vi>, "newStatus"=w1150:bool, "ctlstr"=w1149:refnum<vi>)  [unwired: 1 in, 4 out]
            n202 = property on="Property Node" class="Bool (strict)"(reference=w1151, "Val(Sgnl)"=w1150) -> ()  [unwired: 1 in, 2 out]
            n203 = case shown="\"default\"" w1148 {
              selector: w1148 -> [_ w1152]
              tunnel: w1149 -> [_ w1153]
              frame "default" {
              }
              frame "", Default {
                n204 = property on="Property Node" class="Str"(reference=w1153, "Value"=w1152) -> ()  [unwired: 1 in, 2 out]
              }
            }
          }
          event "clearNotifications": Value Change {
            n205 = event-data() -> ("OldVal"=w1161:bool, "NewVal"=w1160:bool)  [unwired: 1 in, 4 out]
            n206 = Less?(x=w1161, y=w1160) -> (x < y?=w1159:bool)
            n207 = case shown="True" w1159 {
              tunnel: ["" "clearNotifications"] -> w1155
              tunnel: ["gen" "updui"] -> w1154
              frame False {
              }
              frame True {
              }
            }
            n208 = Bundle(w1155, w1154, "Variant"=w1156) -> (w1158:cluster{string, string, "Variant":variant})  [unwired: 1 in]
            n209 = Build Array(w1158) -> (w1157:cluster{string, string, "Variant":variant}[])
          }
          event "initALL": Value Change {
            n210 = event-data() -> ("OldVal"=w1172:bool, "NewVal"=w1171:bool)  [unwired: 1 in, 4 out]
            n211 = control-ref of="initMAT"() -> (w1168:refnum<vi>)
            n212 = control-ref of="initCCD"() -> (w1169:refnum<vi>)
            n213 = control-ref of="initMIL"() -> (w1174:refnum<vi>)
            n214 = control-ref of="initLIA"() -> (w1176:refnum<vi>)
            n215 = control-ref of="initSPT"() -> (w1175:refnum<vi>)
            n216 = Build Array(w1176, w1175, w1174, w1169, w1168) -> (w1173:refnum<vi>[])
            n217 = Less?(x=w1172, y=w1171) -> (x < y?=w1170:bool)
            n218 = case shown="False" w1170 {
              selector: w1170 -> [_ w1186]
              tunnel: [w1184 w1186] -> w1167
              frame False {
                n219 = Two Button Dialog(message="Disconnect all instruments?") -> (T button?=w1184:bool)  [unwired: 2 in]
              }
              frame True {
              }
            }
            n220 = case shown="True" w1167 {
              tunnel: w1173 -> [_ w1179]
              tunnel: w1171 -> [_ w1178]
              tunnel: [_ w1177] -> w1166
              frame False {
              }
              frame True {
                n221 = for {
                  tunnel: w1179 -> [w1183] mode=indexing
                  shift-right: [w1182] -> w1177
                  shift-left: _ -> [w1181]
                  tunnel: w1178 -> [w1180]
                  n222 = property class="Bool (strict)"(reference=w1183, error in=w1181, "Val(Sgnl)"=w1180) -> (error out=w1182:errorcluster)  [unwired: 1 out]
                }
              }
            }
          }
          event User Event {
            n223 = event-data() -> ("elementArr"=w1187:T12)  [unwired: 1 in, 4 out]
          }
          event "initMAT", "initSPT", "initMIL", "initCCD", "initLIA": Value Change {
            w1205 = 3
            # "NOT DONE"
            n224 = event-data() -> ("Source"=w1209:T13, "CtlRef"=w1190:refnum<vi>, "OldVal"=w1189:bool, "NewVal"=w1202:bool)  [unwired: 1 in, 2 out]
            n225 = property class="Bool (strict)"(reference=w1190) -> ("Label.Text"=w1206:string)  [unwired: 1 in, 2 out]
            n226 = String Length(string=w1206) -> (length=w1207:i32)
            n227 = Subtract(x=w1207, y=w1205) -> (x-y=w1204:i32)
            n228 = Greater?(x=w1202, y=w1189) -> (0:w1203:bool)
            n229 = String Subset(string=w1206, offset (0)=w1204, length (rest)=w1205) -> (substring=w1201:string)
            n230 = case shown="False" w1203 {
              tunnel: w1209 -> [_ _]
              tunnel: ["shutdown" "init"] -> w1199
              tunnel: w1201 -> [_ _]
              tunnel: [TRUE TRUE] -> w1200
              tunnel: ["shut down " "initialize "] -> w1192
              frame False {
                # "HERE GOES A\nA VI THAT CHECKS WHETHER\nOR NOT INSTRUMENT CAN BE \nSHUTDOWN/INIT => 1/0"
              }
              frame True {
                # "HERE GOES A\nA VI THAT CHECKS WHETHER\nOR NOT INSTRUMENT CAN BE \nSHUTDOWN/INIT => 1/0"
              }
            }
            n231 = for {
              tunnel: w1208 -> [w1228] mode=indexing
              tunnel: w1201 -> [w1227]
              tunnel: [w1225] -> w1193
              tunnel: [w1224] -> w1188
              stop <- w1226 stop-if-true
              n232 = Unbundle(w1228) -> ("abbrMAT"=w1224:string, "nameMAT"=w1225:string)
              n233 = Equal?(x=w1224, y=w1227) -> (x = y?=w1226:bool)
            }
            n234 = case shown="True" w1200 {
              tunnel: w1199 -> [_ w1218]
              tunnel: ["" w1218] -> w1195
              tunnel: w1193 -> [w1212 w1223]
              tunnel: w1192 -> [w1213 w1221]
              tunnel: [w1216 w1219] -> w1191
              tunnel: w1190 -> [w1211 _]
              tunnel: w1189 -> [w1210 _]
              frame False {
                # "Don't send command."
                n235 = property class="Bool (strict)"(reference=w1211, "Value"=w1210) -> ()  [unwired: 1 in, 2 out]
                n236 = Concatenate Strings("Unable to ", w1213, w1212, ".") -> (w1216:string)
              }
              frame True {
                # "Send command"
                n237 = Concatenate Strings("Beginning to ", w1221, w1223, "...") -> (w1219:string)
              }
            }
            n238 = To Variant(anything=w1193) -> (Variant=w1194:variant)
            n239 = Bundle(w1195, "abbrMAT"=w1188, "Variant"=w1194) -> (w1197:T14)  [unwired: 1 in]
            n240 = Build Array(w1197) -> (w1196:T15)
            n241 = call "writeNotification.vi"("string"=w1191, "Array"=w1198) -> ()  [unwired: 10 in]
          }
          event "Start chopping": Value Change {
            n242 = event-data() -> ("NewVal"=w1235:bool)  [unwired: 1 in, 5 out]
            n243 = To Variant(anything=FALSE) -> (Variant=w1237:variant)
            n244 = To Variant(anything=w1235) -> (Variant=w1243:variant)
            n245 = Bundle("toggleChop", "LIA", "Variant"=w1243) -> (w1242:cluster{string, string, "Variant":variant})  [unwired: 1 in]
            n246 = Bundle("LIAconn", "upduiLIA", "Variant"=w1237) -> (w1236:cluster{string, string, "Variant":variant})  [unwired: 1 in]
            n247 = Build Array(w1242, w1236) -> (w1241:cluster{string, string, "Variant":variant}[])
          }
          event "Chopping Frequency": Value Change {
            n248 = event-data() -> ("NewVal"=w1247:dbl)  [unwired: 1 in, 5 out]
            n249 = local read "Start chopping"() -> (w1246:bool)
            n250 = case shown="True" w1246 {
              tunnel: [_ w1252] -> w1248
              tunnel: w1247 -> [_ w1249]
              frame False {
              }
              frame True {
                n251 = Bundle("NewVal"=w1249, FALSE) -> (w1251:cluster{"NewVal":dbl, bool})  [unwired: 1 in]
                n252 = To Variant(anything=w1251) -> (Variant=w1254:variant)
                n253 = Bundle("setChopFreq", "LIA", "Variant"=w1254) -> (w1253:cluster{string, string, "Variant":variant})  [unwired: 1 in]
                n254 = Build Array(w1253) -> (w1252:cluster{string, string, "Variant":variant}[])
              }
            }
          }
        }
        n255 = case shown="No Error" w1110 {
          tunnel: w1117 -> [w1125 w1135]
          tunnel: w1116 -> [w1124 w1136]
          tunnel: [FALSE TRUE] -> w1115
          tunnel: w1114 -> [w1123 _]
          frame No Error {
            n256 = for {
              tunnel: w1123 -> [w1128] mode=indexing
              tunnel: w1124 -> [w1127]
              shift-right: [w1126] -> _
              shift-left: w1125 -> [w1129]
              stop <- w1126 stop-if-true
              n257 = Enqueue Element(queue=w1127, element=w1128, error in (no error)=w1129) -> (error out=w1126:errorcluster)  [unwired: 1 in, 2 out]
            }
          }
          frame Error {
            n258 = To Variant(anything=0) -> (Variant=w1131:variant)
            n259 = Bundle("Command"="Exit", "Command class"="gen", "Variant"=w1131) -> (w1130:T10)  [unwired: 1 in]
            n260 = Enqueue Element(queue=w1136, element=w1130, error in (no error)=w1135) -> ()  [unwired: 1 in, 3 out]
          }
        }
      }
      n261 = Bundle("command", "command class", variant) -> (w331:cluster{string, string, variant})  [unwired: 1 in]
      n262 = Bundle("command", "command class", variant) -> (w326:cluster{string, string, variant})  [unwired: 1 in]
      n263 = Bundle("command", "command class", variant) -> (w321:cluster{string, string, variant})  [unwired: 1 in]
      n264 = Bundle("command", "command class", variant) -> (w316:cluster{string, string, variant})  [unwired: 1 in]
      n265 = Bundle("command", "command class", variant) -> (w285:cluster{string, string, variant})  [unwired: 1 in]
      n266 = Obtain Queue(name (unnamed)="sptq", element data type=w331) -> (queue out=w274:refnum<queue>, error out=w275:errorcluster)  [unwired: 3 in, 1 out]
      n267 = Obtain Queue(name (unnamed)="ccdq", element data type=w326) -> (queue out=w276:refnum<queue>, error out=w277:errorcluster)  [unwired: 3 in, 1 out]
      n268 = Obtain Queue(name (unnamed)="liaq", element data type=w321) -> (queue out=w278:refnum<queue>, error out=w279:errorcluster)  [unwired: 3 in, 1 out]
      n269 = Obtain Queue(name (unnamed)="matq", element data type=w316) -> (queue out=w280:refnum<queue>, error out=w281:errorcluster)  [unwired: 3 in, 1 out]
      n270 = Obtain Queue(name (unnamed)="uiq", element data type=w285) -> (queue out=w282:refnum<queue>, error out=w283:errorcluster)  [unwired: 3 in, 1 out]
      n271 = Bundle("command", "command class", variant) -> (w311:cluster{string, string, variant})  [unwired: 1 in]
      n272 = Bundle("command", "command class", variant) -> (w306:cluster{string, string, variant})  [unwired: 1 in]
      n273 = Bundle("command", "command class", variant) -> (w301:cluster{string, string, variant})  [unwired: 1 in]
      n274 = Bundle("command", "command class", variant) -> (w296:cluster{string, string, variant})  [unwired: 1 in]
      n275 = Obtain Queue(name (unnamed)="milq", element data type=w311) -> (queue out=w273:refnum<queue>, error out=w272:errorcluster)  [unwired: 3 in, 1 out]
      n276 = Obtain Queue(name (unnamed)="placeholder1", element data type=w306) -> (queue out=w271:refnum<queue>, error out=w270:errorcluster)  [unwired: 3 in, 1 out]
      n277 = Obtain Queue(name (unnamed)="placeholder2", element data type=w301) -> (queue out=w269:refnum<queue>, error out=w268:errorcluster)  [unwired: 3 in, 1 out]
      n278 = Obtain Queue(name (unnamed)="placeholder3", element data type=w296) -> (queue out=w267:refnum<queue>, error out=w266:errorcluster)  [unwired: 3 in, 1 out]
      n279 = while {
        tunnel: w350 -> [w875]
        tunnel: w351 -> [w874]
        tunnel: [w873] -> w358
        tunnel: [w870] -> w360
        tunnel: w262 -> [w866]
        tunnel: w274 -> [w850]
        tunnel: w275 -> [w851]
        tunnel: w276 -> [w852]
        tunnel: w277 -> [w853]
        tunnel: w278 -> [w854]
        tunnel: w279 -> [w855]
        tunnel: w280 -> [w856]
        tunnel: w281 -> [w857]
        tunnel: w273 -> [w858]
        tunnel: w272 -> [w859]
        tunnel: w271 -> [w860]
        tunnel: w270 -> [w861]
        tunnel: w269 -> [w862]
        tunnel: w268 -> [w863]
        tunnel: w267 -> [w864]
        tunnel: w266 -> [w865]
        tunnel: w283 -> [w849]
        tunnel: w282 -> [w848]
        stop <- w869 stop-if-true
        # "DISTRIBUTOR\nAssigns 'mainq' commands to separate queues for each worker\n- operates on 1/16 slave timebase"
        n280 = Dequeue Element(queue=w875, error in (no error)=w874) -> (queue out=w873:refnum<queue>, element=w871:cluster{string, string, variant}, error out=w870:errorcluster)  [unwired: 1 in, 1 out]
        n281 = Unbundle(w871) -> (w872:string)  [unwired: 2 out]
        n282 = case shown="\"MAT\"" w872 {
          tunnel: w871 -> [w876 w881 w884 w887 w890 w893 w896 w898 w899 w902 w905 w908]
          tunnel: w865 -> [_ _ _ _ _ _ _ _ _ _ _ _]
          tunnel: w864 -> [_ _ _ _ _ _ _ w897 _ _ _ _]
          tunnel: w863 -> [_ _ _ _ _ _ w895 _ _ _ _ _]
          tunnel: w862 -> [_ _ _ _ _ _ w894 _ _ _ _ _]
          tunnel: w861 -> [_ _ _ _ _ w892 _ _ _ _ _ _]
          tunnel: w860 -> [_ _ _ _ _ w891 _ _ _ _ _ _]
          tunnel: w859 -> [_ _ _ _ w888 _ _ _ _ _ _ _]
          tunnel: w858 -> [_ _ _ _ w889 _ _ _ _ _ _ _]
          tunnel: w857 -> [_ _ _ w885 _ _ _ _ _ _ _ _]
          tunnel: w856 -> [_ _ _ w886 _ _ _ _ _ _ _ _]
          tunnel: w855 -> [_ _ w882 _ _ _ _ _ _ _ _ _]
          tunnel: w854 -> [_ _ w883 _ _ _ _ _ _ _ _ _]
          tunnel: w853 -> [_ w879 _ _ _ _ _ _ _ _ _ _]
          tunnel: w852 -> [_ w880 _ _ _ _ _ _ _ _ _ _]
          tunnel: w851 -> [w878 _ _ _ _ _ _ _ _ _ _ _]
          tunnel: w850 -> [w877 _ _ _ _ _ _ _ _ _ _ _]
          tunnel: w849 -> [_ _ _ _ _ _ _ _ w901 w904 w907 w910]
          tunnel: w848 -> [_ _ _ _ _ _ _ _ w900 w903 w906 w909]
          frame "SPT" {
            n283 = Enqueue Element(queue=w877, element=w876, error in (no error)=w878) -> ()  [unwired: 1 in, 3 out]
          }
          frame "CCD" {
            n284 = Enqueue Element(queue=w880, element=w881, error in (no error)=w879) -> ()  [unwired: 1 in, 3 out]
          }
          frame "LIA" {
            n285 = Enqueue Element(queue=w883, element=w884, error in (no error)=w882) -> ()  [unwired: 1 in, 3 out]
          }
          frame "MAT" {
            n286 = Enqueue Element(queue=w886, element=w887, error in (no error)=w885) -> ()  [unwired: 1 in, 3 out]
          }
          frame "MIL" {
            n287 = Enqueue Element(queue=w889, element=w890, error in (no error)=w888) -> ()  [unwired: 1 in, 3 out]
          }
          frame "placeholder1" {
            n288 = Enqueue Element(queue=w891, element=w893, error in (no error)=w892) -> ()  [unwired: 1 in, 3 out]
          }
          frame "placeholder2" {
            n289 = Enqueue Element(queue=w894, element=w896, error in (no error)=w895) -> ()  [unwired: 1 in, 3 out]
          }
          frame "placeholder3" {
            n290 = Enqueue Element(queue=w897, element=w898) -> ()  [unwired: 2 in, 3 out]
          }
          frame "gen", Default {
            n291 = Enqueue Element(queue=w900, element=w899, error in (no error)=w901) -> ()  [unwired: 1 in, 3 out]
          }
          frame "updui" {
            n292 = Enqueue Element(queue=w903, element=w902, error in (no error)=w904) -> ()  [unwired: 1 in, 3 out]
          }
          frame "upduiLIA" {
            n293 = Enqueue Element(queue=w906, element=w905, error in (no error)=w907) -> ()  [unwired: 1 in, 3 out]
          }
          frame "disb" {
            n294 = Enqueue Element(queue=w909, element=w908, error in (no error)=w910) -> ()  [unwired: 1 in, 3 out]
          }
        }
        n295 = Unbundle By Name(w870) -> ("status"=w869:bool)
        n296 = Scale By Power Of 2(n=-4, x=w866) -> (x*2^n=w867:dbl)
        n297 = Wait Until Next ms Multiple(millisecond multiple=w867) -> ()  [unwired: 1 out]
      }
      n298 = Release Queue(queue=w358, error in (no error)=w360) -> (error out=w357:errorcluster)  [unwired: 3 out]
      n299 = call <vilib>:"Simple Error Handler.vi"("error in (no error)"=w357) -> ()  [unwired: 1 in, 8 out]
      n300 = while {
        tunnel: [w965] -> w366
        tunnel: w283 -> [w960]
        tunnel: w282 -> [w961]
        tunnel: [w964] -> w365
        tunnel: w258 -> [w951]
        tunnel: w262 -> [w952]
        tunnel: w259 -> [w950]
        stop <- w949 stop-if-true
        # "Current command classes:\ngen, updui, disb"
        # "WORKER I\nExecute upon 'mainq' commands\n - operates on 1/8 slave timebase"
        n301 = Get Queue Status(queue=w961, error in (no error)=w960) -> (queue out=w964:refnum<queue>, error out=w965:errorcluster)  [unwired: 7 out]
        n302 = Dequeue Element(queue=w961, error in (no error)=w960) -> (queue out=w956:refnum<queue>, element=w955:cluster{string, string, variant}, error out=w963:errorcluster)  [unwired: 1 in, 1 out]
        n303 = Unbundle(w955) -> (w962:string, w958:string, w957:variant)
        n304 = case shown="\"upduiLIA\"" w958 {
          tunnel: w963 -> [w971 w993 w1033 w1072 w1102 w1107]
          tunnel: w962 -> [w968 w991 w1031 w1070 w1099 _]
          tunnel: [w970 FALSE FALSE FALSE w1101 FALSE] -> _
          tunnel: [w969 w992 w1032 w1071 w1100 ""] -> w959
          tunnel: w957 -> [_ w988 w1028 w1067 _ _]
          tunnel: w956 -> [_ _ _ _ _ w1109]
          tunnel: w955 -> [_ _ _ _ _ w1108]
          tunnel: w951 -> [w966 w989 w1029 w1068 w1097 _]
          tunnel: w950 -> [w967 w990 w1030 w1069 w1098 _]
          frame "gen" {
            n305 = case shown="\"Init\"" w968 {
              tunnel: w971 -> [_ _ _ _]
              tunnel: [FALSE FALSE TRUE FALSE] -> w970
              tunnel: ["" "Stopping..." "Closing down..." "Initializing interface..."] -> w969
              tunnel: w967 -> [_ _ _ w980]
              tunnel: w966 -> [_ _ _ w982]
              frame Default {
              }
              frame "BeginStop" {
              }
              frame "Exit" {
              }
              frame "Init" {
                n306 = call "UIinitializationCommands.vi"() -> ("array of cmds"=w984:T16)  [unwired: 2 in]
                n307 = Unbundle(w980) -> (w979:T4, w978:cluster{string, "qintoMain":refnum<user-event>})
                n308 = call "changeLED_event.vi"("eventcluster"=w979, "LED?"="GUI-busy", "newStatus"=TRUE, "ctlarr"=w982) -> ()  [unwired: 9 in, 3 out]
                n309 = call "enqMulti.vi"("array of cmds"=w984, "eventcluster"=w978) -> ()  [unwired: 9 in, 1 out]
              }
            }
          }
          frame "updui" {
            n310 = case shown="\"InitFin\"" w991 {
              tunnel: w993 -> [_ _ _ w1006 _]
              tunnel: ["" w995 "Notifications cleared." "Interface initialization complete." _] -> w992
              tunnel: w990 -> [_ _ _ w1010 w1021]
              tunnel: w989 -> [_ w996 _ w1001 w1022]
              tunnel: w988 -> [_ w997 _ _ w1026]
              frame Default {
                (unwired) FALSE
              }
              frame "setPowerLim" {
                n311 = call "setPowerLim.vi"("ctlref"=w996, "Variant"=w997) -> ("notification"=w995:string)
              }
              frame "clearNotifications" {
                n312 = control-ref of="Notifications"() -> (w1000:refnum<vi>)
                n313 = property class="Str"(reference=w1000, "Value"="") -> ()  [unwired: 1 in, 2 out]
              }
              frame "InitFin" {
                n314 = Unbundle(w1010) -> (w1007:T4)  [unwired: 1 out]
                n315 = call "changeLED_event.vi"("eventcluster"=w1007, "LED?"="GUI-busy", "newStatus"=FALSE, "ctlarr"=w1001, "error in (no error)"=w1006) -> ("eventclusterOut"=w1005:T17, "ctlarrOut"=w1004:T9, "error out"=w1003:errorcluster)  [unwired: 8 in]
                n316 = call "getInstrAbbr.vi"("ctlarr"=w1001) -> ("abbrArray"=w1002:string[])
                n317 = for {
                  tunnel: w1005 -> [w1016]
                  tunnel: w1004 -> [w1015]
                  tunnel: w1003 -> [w1014]
                  tunnel: w1002 -> [w1019] mode=indexing
                  n318 = Concatenate Strings(w1019, "-status") -> (w1017:string)
                  n319 = call "changeLED_event.vi"("eventcluster"=w1016, "LED?"=w1017, "string?"="Disconnected", "newStatus"=FALSE, "ctlarr"=w1015, "error in (no error)"=w1014) -> ()  [unwired: 7 in, 3 out]
                }
              }
              frame "LIAconn" {
                n320 = Variant To Data(type=TRUE, Variant=w1026) -> (data=w1024:bool)  [unwired: 1 in, 1 out]
                n321 = Unbundle(w1021) -> (w1020:T4)  [unwired: 1 out]
                n322 = call "changeLED_event.vi"("eventcluster"=w1020, "LED?"="LIA-status", "newStatus"=w1024, "ctlarr"=w1022) -> ()  [unwired: 9 in, 3 out]
              }
            }
          }
          frame "upduiLIA" {
            n323 = case shown="Default" w1031 {
              tunnel: w1033 -> [_ _ _ _]
              tunnel: ["" _ _ _] -> w1032
              tunnel: w1030 -> [_ w1036 w1043 w1060]
              tunnel: w1029 -> [_ w1037 w1045 w1061]
              tunnel: w1028 -> [_ w1041 w1044 _]
              frame Default {
                (unwired) FALSE
              }
              frame "LIAconn" {
                n324 = Variant To Data(type=TRUE, Variant=w1041) -> (data=w1039:bool)  [unwired: 1 in, 1 out]
                n325 = Unbundle(w1036) -> (w1035:T4)  [unwired: 1 out]
                n326 = call "changeLED_event.vi"("eventcluster"=w1035, "LED?"="LIA-status", "newStatus"=w1039, "ctlarr"=w1037) -> ()  [unwired: 9 in, 3 out]
              }
              frame "writeStrCHOP" {
                n327 = local read "Start chopping"() -> (w1042:bool)
                n328 = case shown="True" w1042 {
                  tunnel: w1045 -> [_ w1052]
                  tunnel: w1044 -> [_ w1051]
                  tunnel: w1043 -> [_ w1048]
                  frame False {
                  }
                  frame True {
                    n329 = Variant To Data(type=0, Variant=w1051) -> (data=w1049:i32)  [unwired: 1 in, 1 out]
                    n330 = Unbundle(w1048) -> (w1047:T4)  [unwired: 1 out]
                    n331 = Number To Decimal String(number=w1049) -> (decimal integer string=w1057:string)  [unwired: 1 in]
                    n332 = local read "connLIA"() -> (w1053:bool)
                    n333 = Concatenate Strings("Chop at ", w1057, " Hz...") -> (w1058:string)
                    n334 = local write "LIAtimer1"(TRUE) -> ()
                    n335 = call "changeLED_event.vi"("eventcluster"=w1047, "LED?"="LIA-conn", "string?"=w1058, "newStatus"=w1053, "ctlarr"=w1052) -> ()  [unwired: 8 in, 3 out]
                  }
                }
              }
              frame "writeStrIDLE" {
                n336 = Unbundle(w1060) -> (w1065:T4)  [unwired: 1 out]
                n337 = local read "connLIA"() -> (w1059:bool)
                n338 = call "changeLED_event.vi"("eventcluster"=w1065, "LED?"="LIA-conn", "string?"="Idle", "newStatus"=w1059, "ctlarr"=w1061) -> ()  [unwired: 8 in, 3 out]
                n339 = local write "LIAtimer1"(FALSE) -> ()
              }
            }
          }
          frame "disb" {
            n340 = case shown="\"toggleVISAfields\"" w1070 {
              tunnel: w1072 -> [_ _ w1076 w1086 w1095]
              tunnel: ["" _ _ _ _] -> w1071
              tunnel: w1069 -> [_ _ _ _ _]
              tunnel: w1068 -> [_ w1075 w1079 w1088 w1096]
              tunnel: w1067 -> [_ w1074 w1078 w1085 w1094]
              frame Default {
                (unwired) FALSE
              }
              frame "toggleInstrSett" {
                n341 = call "toggleCtlVis.vi"("ctlarr"=w1075, "Variant"=w1074) -> ()  [unwired: 8 in, 2 out]
              }
              frame "toggleVISAfields" {
                n342 = call "toggleCtlVis.vi"("error in (no error)"=w1076, "ctlarr"=w1079, "Variant"=w1078, "tag?"="visa") -> ()  [unwired: 6 in, 2 out]
              }
              frame "visLIApanelVISA" {
                n343 = Variant To Data(type=TRUE, Variant=w1085) -> (data=w1082:bool)  [unwired: 1 in, 1 out]
                n344 = Bundle("LIA", w1082) -> (w1081:cluster{string, bool})  [unwired: 1 in]
                n345 = To Variant(anything=w1081) -> (Variant=w1080:variant)
                n346 = call "toggleCtlVis.vi"("error in (no error)"=w1086, "ctlarr"=w1088, "Variant"=w1080, "tag?"="visa") -> ()  [unwired: 6 in, 2 out]
              }
              frame "visLIApanel" {
                n347 = Variant To Data(type=TRUE, Variant=w1094) -> (data=w1091:bool)  [unwired: 1 in, 1 out]
                n348 = Bundle("LIA", w1091) -> (w1090:cluster{string, bool})  [unwired: 1 in]
                n349 = To Variant(anything=w1090) -> (Variant=w1089:variant)
                n350 = call "toggleCtlVis.vi"("error in (no error)"=w1095, "ctlarr"=w1096, "Variant"=w1089) -> ()  [unwired: 7 in, 2 out]
              }
            }
          }
          frame "placeholder" {
            n351 = case shown="Default" w1099 {
              tunnel: w1102 -> [_]
              tunnel: [FALSE] -> w1101
              tunnel: [""] -> w1100
              tunnel: w1098 -> [_]
              tunnel: w1097 -> [_]
              frame Default {
              }
            }
          }
          frame Default {
            n352 = Enqueue Element(queue=w1109, element=w1108, error in (no error)=w1107) -> ()  [unwired: 1 in, 3 out]
          }
        }
        n353 = Unbundle By Name(w965) -> ("status"=w949:bool)
        n354 = Scale By Power Of 2(n=-3, x=w952) -> (x*2^n=w953:dbl)
        n355 = Wait Until Next ms Multiple(millisecond multiple=w953) -> ()  [unwired: 1 out]
        n356 = call "writeNotification.vi"("string"=w959, "Array"=w951) -> ()  [unwired: 10 in]
      }
      n357 = while {
        tunnel: [w929] -> w361
        tunnel: w275 -> [w925]
        tunnel: w274 -> [w926]
        tunnel: w258 -> [w914]
        tunnel: w262 -> [w916]
        tunnel: [w915] -> w362
        tunnel: w259 -> [w913]
        shift-right: [w911] -> _
        shift-left: w264 -> [w912]
        stop <- w917 stop-if-true
        # "[SPT] WORKER II \nExecute upon 'mainq' commands\n - operates on slave timebase"
        n358 = Get Queue Status(queue=w926, error in (no error)=w925) -> (queue out=w915:refnum<queue>, error out=w929:errorcluster)  [unwired: 7 out]
        n359 = Dequeue Element(queue=w926, error in (no error)=w925) -> (queue out=w921:refnum<queue>, element=w920:cluster{string, string, variant}, error out=w928:errorcluster)  [unwired: 1 in, 1 out]
        n360 = Unbundle(w920) -> (w927:string, w923:string, w922:variant)
        n361 = case shown="\"SPT\"" w923 {
          tunnel: w928 -> [w935 w942 w946]
          tunnel: w927 -> [w933 w940 _]
          tunnel: [w934 w941 ""] -> w924
          tunnel: w922 -> [w931 w938 _]
          tunnel: w921 -> [_ _ w948]
          tunnel: w920 -> [_ _ w947]
          tunnel: w914 -> [w932 w939 _]
          tunnel: w913 -> [_ _ _]
          tunnel: w912 -> [w930 w937 w944]
          tunnel: [w930 w937 w944] -> w911
          frame "SPT" {
            n362 = case shown="Default" w933 {
              tunnel: w935 -> [_]
              tunnel: [""] -> w934
              tunnel: w932 -> [_]
              tunnel: w931 -> [_]
              frame Default {
              }
            }
          }
          frame "placeholder" {
            n363 = case shown="Default" w940 {
              tunnel: w942 -> [_]
              tunnel: [""] -> w941
              tunnel: w939 -> [_]
              tunnel: w938 -> [_]
              frame Default {
              }
            }
          }
          frame Default {
            n364 = Enqueue Element(queue=w948, element=w947, error in (no error)=w946) -> ()  [unwired: 1 in, 3 out]
          }
        }
        n365 = Unbundle By Name(w929) -> ("status"=w917:bool)
        n366 = Scale By Power Of 2(n=0, x=w916) -> (x*2^n=w918:dbl)
        n367 = Wait Until Next ms Multiple(millisecond multiple=w918) -> ()  [unwired: 1 out]
        n368 = call "writeNotification.vi"("string"=w924, "Array"=w914) -> ()  [unwired: 10 in]
      }
      n369 = while {
        tunnel: [w596] -> w345
        tunnel: w279 -> [w592]
        tunnel: w278 -> [w593]
        tunnel: w258 -> [w581]
        tunnel: w262 -> [w583]
        tunnel: [w582] -> w346
        tunnel: w259 -> [w580]
        shift-right: [w578] -> _
        shift-left: w264 -> [w579]
        tunnel: w264 -> [w577]
        stop <- w584 stop-if-true
        # "Current commands:\ninit, shutdown"
        # "[LIA] WORKER IV\nExecute upon 'mainq' commands\n - operates on slave timebase"
        n370 = Dequeue Element(queue=w593, error in (no error)=w592) -> (queue out=w588:refnum<queue>, element=w587:cluster{string, string, variant}, error out=w595:errorcluster)  [unwired: 1 in, 1 out]
        n371 = Get Queue Status(queue=w593, error in (no error)=w592) -> (queue out=w582:refnum<queue>, error out=w596:errorcluster)  [unwired: 7 out]
        n372 = Unbundle(w587) -> (w594:string, w590:string, w589:variant)
        n373 = case shown="\"LIA\"" w590 {
          tunnel: w595 -> [w605 w786 w791]
          tunnel: w594 -> [w603 w784 _]
          tunnel: [w604 w785 ""] -> w591
          tunnel: w589 -> [w601 w782 _]
          tunnel: w588 -> [_ _ w793]
          tunnel: w587 -> [_ _ w792]
          tunnel: w581 -> [w602 w783 _]
          tunnel: w580 -> [w598 _ _]
          tunnel: w579 -> [w600 w781 w789]
          tunnel: [w599 w780 w789] -> w578
          tunnel: w577 -> [w597 _ _]
          frame "LIA" {
            n374 = case shown="\"init\"" w603 {
              tunnel: w605 -> [_ _ _ _ _]
              tunnel: ["" w609 w663 _ _] -> w604
              tunnel: w602 -> [_ w611 w665 w709 _]
              tunnel: w601 -> [_ _ _ w713 w747]
              tunnel: w600 -> [w606 _ w662 w711 w754]
              tunnel: [w606 w612 w666 w710 w750] -> w599
              tunnel: w598 -> [_ w610 w664 w708 w752]
              tunnel: w597 -> [_ w608 w661 w712 _]
              frame Default {
              }
              frame "init" {
                n375 = stacked-sequence {
                  seq-local: [w614 _ _] -> [_ w630 w644]
                  tunnel: [w615 _ _] -> w612
                  tunnel: w611 -> [_ _ w645]
                  tunnel: w610 -> [_ w629 w647]
                  tunnel: [_ _ w643] -> w609
                  tunnel: w608 -> [w613 _ _]
                  frame #0 {
                    n376 = local read "actDummy"() -> (w616:bool)
                    n377 = local read "visaLIA"() -> (w617:string)
                    n378 = case shown="False" w616 {
                      tunnel: w617 -> [w625 _]
                      tunnel: [w620 w626] -> w615
                      tunnel: [w621 w627] -> w614
                      tunnel: w613 -> [_ w626]
                      frame False {
                        n379 = call <instrlib>:"Initialize.vi"("VISA resource name"=w625) -> ("error out"=w624:errorcluster, "VISA resource name out"=w623:refnum<visa-resource-name>)  [unwired: 9 in]
                        n380 = call <instrlib>:"Configure Chopper.vi"("error in (no error)"=w624, "Chopper Blade (0: 6-slot)"=1, "VISA resource name"=w623) -> ("error out"=w622:errorcluster, "VISA resource name out"=w619:refnum<visa-resource-name>)  [unwired: 7 in]
                        n381 = call "InitializeChop.vi"("error in (no error)"=w622, "VISA resource name"=w619) -> ("error out"=w621:errorcluster, "VISA resource name out"=w620:refnum<visa-resource-name>)  [unwired: 8 in]
                      }
                      frame True {
                        n382 = xnode "Error Ring"() -> ("error out"=w627:errorcluster)
                      }
                    }
                  }
                  frame #1 {
                    n383 = case shown="No Error" w630 {
                      tunnel: w629 -> [w632 _]
                      frame No Error {
                        w636 = "disb"
                        n384 = Unbundle(w632) -> (w631:cluster{string, "qintoMain":refnum<user-event>})  [unwired: 1 out]
                        n385 = To Variant(anything=TRUE) -> (Variant=w639:variant)
                        n386 = To Variant(anything=FALSE) -> (Variant=w640:variant)
                        n387 = Bundle("visLIApanel", w636, "Variant"=w639) -> (w635:cluster{string, string, "Variant":variant})  [unwired: 1 in]
                        n388 = Bundle("visLIApanelVISA", w636, "Variant"=w640) -> (w634:cluster{string, string, "Variant":variant})  [unwired: 1 in]
                        n389 = Build Array(w635, w634) -> (w633:cluster{string, string, "Variant":variant}[])
                        n390 = call "enqMulti.vi"("array of cmds"=w633, "eventcluster"=w631) -> ()  [unwired: 9 in, 1 out]
                      }
                      frame Error {
                      }
                    }
                  }
                  frame #2 {
                    n391 = Unbundle(w647) -> (w646:T4)  [unwired: 1 out]
                    n392 = case shown="No Error" w644 {
                      selector: w644 -> [w656 _]
                      tunnel: w645 -> [w655 _]
                      tunnel: w646 -> [w653 _]
                      tunnel: [w649 w658] -> w643
                      frame No Error {
                        n393 = local read "nameLIA"() -> (w651:string)
                        n394 = call "changeLED_event.vi"("eventcluster"=w653, "LED?"="LIA-conn", "string?"="Idle", "newStatus"=TRUE, "ctlarr"=w655, "error in (no error)"=w656) -> ()  [unwired: 7 in, 3 out]
                        n395 = Concatenate Strings(w651, " connected.") -> (w649:string)
                      }
                      frame Error {
                        n396 = local read "nameLIA"() -> (w660:string)
                        n397 = Concatenate Strings(w660, " could not be connected.") -> (w658:string)
                        n398 = local write "initLIA"(FALSE) -> ()
                      }
                    }
                  }
                }
              }
              frame "shutdown" {
                n399 = stacked-sequence {
                  seq-local: [w669 _ _] -> [_ w677 w691]
                  tunnel: [w667 _ _] -> w666
                  tunnel: w665 -> [_ w676 w692]
                  tunnel: w664 -> [_ w675 w694]
                  tunnel: [_ _ w690] -> w663
                  tunnel: w662 -> [w668 _ _]
                  tunnel: w661 -> [w667 _ _]
                  frame #0 {
                    n400 = local read "actDummy"() -> (w670:bool)
                    n401 = case shown="False" w670 {
                      tunnel: [w672 w673] -> w669
                      tunnel: w668 -> [w671 _]
                      frame False {
                        n402 = call <instrlib>:"Close.vi"("VISA resource name"=w671) -> ("error out"=w672:errorcluster)  [unwired: 10 in]
                      }
                      frame True {
                        n403 = xnode "Error Ring"() -> ("error out"=w673:errorcluster)
                      }
                    }
                  }
                  frame #1 {
                    n404 = case shown="No Error" w677 {
                      tunnel: w676 -> [_ _]
                      tunnel: w675 -> [w678 _]
                      frame No Error {
                        w683 = "disb"
                        n405 = Unbundle(w678) -> (w679:cluster{string, "qintoMain":refnum<user-event>})  [unwired: 1 out]
                        n406 = To Variant(anything=FALSE) -> (Variant=w686:variant)
                        n407 = To Variant(anything=TRUE) -> (Variant=w687:variant)
                        n408 = Bundle("visLIApanel", w683, "Variant"=w686) -> (w682:cluster{string, string, "Variant":variant})  [unwired: 1 in]
                        n409 = Bundle("visLIApanelVISA", w683, "Variant"=w687) -> (w681:cluster{string, string, "Variant":variant})  [unwired: 1 in]
                        n410 = Build Array(w682, w681) -> (w680:cluster{string, string, "Variant":variant}[])
                        n411 = call "enqMulti.vi"("array of cmds"=w680, "eventcluster"=w679) -> ()  [unwired: 9 in, 1 out]
                      }
                      frame Error {
                      }
                    }
                  }
                  frame #2 {
                    n412 = Unbundle(w694) -> (w693:T4)  [unwired: 1 out]
                    n413 = case shown="No Error" w691 {
                      selector: w691 -> [w703 _]
                      tunnel: w692 -> [w702 _]
                      tunnel: w693 -> [w700 _]
                      tunnel: [w696 w705] -> w690
                      frame No Error {
                        n414 = local read "nameLIA"() -> (w698:string)
                        n415 = call "changeLED_event.vi"("eventcluster"=w700, "LED?"="LIA-conn", "string?"="Disconnected", "newStatus"=FALSE, "ctlarr"=w702, "error in (no error)"=w703) -> ()  [unwired: 7 in, 3 out]
                        n416 = Concatenate Strings(w698, " disconnected.") -> (w696:string)
                      }
                      frame Error {
                        n417 = local read "nameLIA"() -> (w707:string)
                        n418 = Concatenate Strings(w707, " could not be connected.") -> (w705:string)
                        n419 = local write "initLIA"(TRUE) -> ()
                      }
                    }
                  }
                }
              }
              frame "setChopFreq" {
                n420 = stacked-sequence {
                  seq-local: [w719 _] -> [_ w737]
                  seq-local: [w715 _] -> [_ w735]
                  tunnel: w713 -> [w724 _]
                  tunnel: w712 -> [w723 _]
                  tunnel: w711 -> [w722 _]
                  tunnel: [w721 _] -> w710
                  tunnel: w709 -> [w718 _]
                  tunnel: w708 -> [_ w738]
                  frame #0 {
                    n421 = local read "actDummy"() -> (w720:bool)
                    n422 = Variant To Data(type=cluster{dbl, bool} {0.0, FALSE} ("output cluster"), Variant=w724) -> (data=w716:cluster{dbl, bool})  [unwired: 1 in, 1 out]
                    n423 = Unbundle(w716) -> (w715:dbl, w714:bool)
                    n424 = case shown="False" w720 {
                      tunnel: w723 -> [w726 _]
                      tunnel: w722 -> [w728 w733]
                      tunnel: [w729 w733] -> w721
                      tunnel: w715 -> [w727 _]
                      tunnel: [w730 w732] -> w719
                      tunnel: w718 -> [w731 _]
                      tunnel: w714 -> [w725 _]
                      frame False {
                        n425 = call "setChopFreq.vi"("arrayIn"=w731, "startup?"=w725, "emptyVISA"=w726, "newfreq"=w727, "VISA resource name"=w728) -> ("error out"=w730:errorcluster, "VISA resource name out"=w729:refnum<visa-resource-name>)  [unwired: 4 in, 1 out]
                      }
                      frame True {
                        n426 = xnode "Error Ring"() -> ("error out"=w732:errorcluster)
                      }
                    }
                  }
                  frame #1 {
                    n427 = Unbundle(w738) -> (w736:cluster{string, "qintoMain":refnum<user-event>})  [unwired: 1 out]
                    n428 = case shown="No Error" w737 {
                      tunnel: w736 -> [w745 _]
                      tunnel: w735 -> [w741 _]
                      frame No Error {
                        n429 = To Variant(anything=w741) -> (Variant=w742:variant)
                        n430 = Bundle("writeStrCHOP", "upduiLIA", "Variant"=w742) -> (w740:cluster{string, string, "Variant":variant})  [unwired: 1 in]
                        n431 = Build Array(w740) -> (w739:cluster{string, string, "Variant":variant}[])
                        n432 = call "enqMulti.vi"("array of cmds"=w739, "eventcluster"=w745) -> ()  [unwired: 9 in, 1 out]
                      }
                      frame Error {
                      }
                    }
                  }
                }
              }
              frame "toggleChop" {
                n433 = Variant To Data(type=TRUE, Variant=w747) -> (data=w746:bool)  [unwired: 1 in, 1 out]
                n434 = local read "actDummy"() -> (w749:bool)
                n435 = Unbundle(w752) -> (w751:cluster{string, "qintoMain":refnum<user-event>})  [unwired: 1 out]
                n436 = case shown="False" w749 {
                  tunnel: w754 -> [w758 w768]
                  tunnel: [w756 w767] -> w753
                  tunnel: [w757 w768] -> w750
                  tunnel: w746 -> [w755 _]
                  frame False {
                    n437 = case shown="True" w755 {
                      tunnel: w758 -> [w761 w765]
                      tunnel: [w760 w764] -> w756
                      tunnel: [w759 w763] -> w757
                      frame True {
                        n438 = call "sendCMD.vi"("Command"="RSRC CHOP", "VISA resource name"=w761) -> ("error out"=w760:errorcluster, "VISA resource name out"=w759:refnum<visa-resource-name>)  [unwired: 7 in, 1 out]
                      }
                      frame False {
                        n439 = call "sendCMD.vi"("Command"="RSRC INT", "VISA resource name"=w765) -> ("error out"=w764:errorcluster, "VISA resource name out"=w763:refnum<visa-resource-name>)  [unwired: 7 in, 1 out]
                      }
                    }
                  }
                  frame True {
                    n440 = xnode "Error Ring"() -> ("error out"=w767:errorcluster)
                  }
                }
                n441 = case shown="No Error" w753 {
                  tunnel: w751 -> [w777 _]
                  tunnel: w746 -> [w771 _]
                  frame No Error {
                    n442 = local read "Chopping Frequency"() -> (w772:dbl)
                    n443 = case shown="False" w771 {
                      tunnel: ["writeStrCHOP" "writeStrIDLE"] -> w770
                      frame True {
                      }
                      frame False {
                      }
                    }
                    n444 = To Variant(anything=w772) -> (Variant=w775:variant)
                    n445 = Bundle(w770, "upduiLIA", "Variant"=w775) -> (w774:cluster{string, string, "Variant":variant})  [unwired: 1 in]
                    n446 = Build Array(w774) -> (w773:cluster{string, string, "Variant":variant}[])
                    n447 = call "enqMulti.vi"("array of cmds"=w773, "eventcluster"=w777) -> ()  [unwired: 9 in, 1 out]
                  }
                  frame Error {
                  }
                }
              }
            }
          }
          frame "placeholder" {
            n448 = case shown="Default" w784 {
              tunnel: w786 -> [_]
              tunnel: [""] -> w785
              tunnel: w783 -> [_]
              tunnel: w782 -> [_]
              tunnel: w781 -> [w787]
              tunnel: [w787] -> w780
              frame Default {
              }
            }
          }
          frame Default {
            n449 = Enqueue Element(queue=w793, element=w792, error in (no error)=w791) -> ()  [unwired: 1 in, 3 out]
          }
        }
        n450 = Unbundle By Name(w596) -> ("status"=w584:bool)
        n451 = Scale By Power Of 2(n=0, x=w583) -> (x*2^n=w585:dbl)
        n452 = Wait Until Next ms Multiple(millisecond multiple=w585) -> ()  [unwired: 1 out]
        n453 = call "writeNotification.vi"("string"=w591, "Array"=w581) -> ()  [unwired: 10 in]
      }
      n454 = while {
        tunnel: [w426] -> w291
        tunnel: w281 -> [w422]
        tunnel: w280 -> [w423]
        tunnel: w258 -> [w411]
        tunnel: w262 -> [w413]
        tunnel: [w412] -> w289
        tunnel: w259 -> [w410]
        shift-right: [w408] -> _
        shift-left: w264 -> [w409]
        stop <- w414 stop-if-true
        # "[MAT] WORKER V\nExecute upon 'mainq' commands\n - operates on slave timebase"
        n455 = Get Queue Status(queue=w423, error in (no error)=w422) -> (queue out=w412:refnum<queue>, error out=w426:errorcluster)  [unwired: 7 out]
        n456 = Dequeue Element(queue=w423, error in (no error)=w422) -> (queue out=w418:refnum<queue>, element=w417:cluster{string, string, variant}, error out=w425:errorcluster)  [unwired: 1 in, 1 out]
        n457 = Unbundle(w417) -> (w424:string, w420:string, w419:variant)
        n458 = case shown="\"MAT\"" w420 {
          tunnel: w425 -> [w432 w439 w443]
          tunnel: w424 -> [w430 w437 _]
          tunnel: [w431 w438 ""] -> w421
          tunnel: w419 -> [w428 w435 _]
          tunnel: w418 -> [_ _ w445]
          tunnel: w417 -> [_ _ w444]
          tunnel: w411 -> [w429 w436 _]
          tunnel: w410 -> [_ _ _]
          tunnel: w409 -> [w427 w434 w441]
          tunnel: [w427 w434 w441] -> w408
          frame "MAT" {
            n459 = case shown="Default" w430 {
              tunnel: w432 -> [_]
              tunnel: [""] -> w431
              tunnel: w429 -> [_]
              tunnel: w428 -> [_]
              frame Default {
              }
            }
          }
          frame "placeholder" {
            n460 = case shown="Default" w437 {
              tunnel: w439 -> [_]
              tunnel: [""] -> w438
              tunnel: w436 -> [_]
              tunnel: w435 -> [_]
              frame Default {
              }
            }
          }
          frame Default {
            n461 = Enqueue Element(queue=w445, element=w444, error in (no error)=w443) -> ()  [unwired: 1 in, 3 out]
          }
        }
        n462 = Unbundle By Name(w426) -> ("status"=w414:bool)
        n463 = Scale By Power Of 2(n=0, x=w413) -> (x*2^n=w415:dbl)
        n464 = Wait Until Next ms Multiple(millisecond multiple=w415) -> ()  [unwired: 1 out]
        n465 = call "writeNotification.vi"("string"=w421, "Array"=w411) -> ()  [unwired: 10 in]
      }
      n466 = while {
        tunnel: [w812] -> w348
        tunnel: w277 -> [w808]
        tunnel: w276 -> [w809]
        tunnel: w258 -> [w797]
        tunnel: w262 -> [w799]
        tunnel: [w798] -> w349
        tunnel: w259 -> [w796]
        shift-right: [w794] -> _
        shift-left: w264 -> [w795]
        stop <- w800 stop-if-true
        # "[CCD] WORKER III \nExecute upon 'mainq' commands\n - operates on slave timebase"
        n467 = Get Queue Status(queue=w809, error in (no error)=w808) -> (queue out=w798:refnum<queue>, error out=w812:errorcluster)  [unwired: 7 out]
        n468 = Dequeue Element(queue=w809, error in (no error)=w808) -> (queue out=w804:refnum<queue>, element=w803:cluster{string, string, variant}, error out=w811:errorcluster)  [unwired: 1 in, 1 out]
        n469 = Unbundle(w803) -> (w810:string, w806:string, w805:variant)
        n470 = case shown="\"CCD\"" w806 {
          tunnel: w811 -> [w818 w825 w829]
          tunnel: w810 -> [w816 w823 _]
          tunnel: [w817 w824 ""] -> w807
          tunnel: w805 -> [w814 w821 _]
          tunnel: w804 -> [_ _ w831]
          tunnel: w803 -> [_ _ w830]
          tunnel: w797 -> [w815 w822 _]
          tunnel: w796 -> [_ _ _]
          tunnel: w795 -> [w813 w820 w827]
          tunnel: [w813 w820 w827] -> w794
          frame "CCD" {
            n471 = case shown="Default" w816 {
              tunnel: w818 -> [_]
              tunnel: [""] -> w817
              tunnel: w815 -> [_]
              tunnel: w814 -> [_]
              frame Default {
              }
            }
          }
          frame "placeholder" {
            n472 = case shown="Default" w823 {
              tunnel: w825 -> [_]
              tunnel: [""] -> w824
              tunnel: w822 -> [_]
              tunnel: w821 -> [_]
              frame Default {
              }
            }
          }
          frame Default {
            n473 = Enqueue Element(queue=w831, element=w830, error in (no error)=w829) -> ()  [unwired: 1 in, 3 out]
          }
        }
        n474 = Unbundle By Name(w812) -> ("status"=w800:bool)
        n475 = Scale By Power Of 2(n=0, x=w799) -> (x*2^n=w801:dbl)
        n476 = Wait Until Next ms Multiple(millisecond multiple=w801) -> ()  [unwired: 1 out]
        n477 = call "writeNotification.vi"("string"=w807, "Array"=w797) -> ()  [unwired: 10 in]
      }
      n478 = Unregister For Events(event registration refnum=w364, error in=w356) -> (error out=w353:errorcluster)
      n479 = case shown="True" FALSE {
        tunnel: w259 -> [_ w837]
        tunnel: [w832 w836] -> w354
        tunnel: w353 -> [w832 _]
        frame False {
        }
        frame True {
          n480 = Unbundle(w837) -> (w835:T4, w834:cluster{string, "qintoMain":refnum<user-event>})
          n481 = for {
            N: 2 -> [_]
            tunnel: [w840] -> w836
            tunnel: w835 -> [w839]
            tunnel: w834 -> [w838]
            i -> [w841]
            n482 = case shown="1" w841 {
              tunnel: [w844 w847] -> w840
              tunnel: w839 -> [w843 _]
              tunnel: w838 -> [_ w845]
              frame 0, Default {
                n483 = Unbundle(w843) -> ("chgStatusLED"=w842:refnum<user-event>)  [unwired: 1 out]
                n484 = Destroy User Event(user event=w842) -> (error out=w844:errorcluster)  [unwired: 1 in]
              }
              frame 1 {
                n485 = Unbundle(w845) -> ("qintoMain"=w846:refnum<user-event>)  [unwired: 1 out]
                n486 = Destroy User Event(user event=w846) -> (error out=w847:errorcluster)  [unwired: 1 in]
              }
            }
          }
        }
      }
      n487 = Release Queue(queue=w289, error in (no error)=w291) -> (error out=w290:errorcluster)  [unwired: 3 out]
      n488 = Release Queue(queue=w362, error in (no error)=w361) -> (error out=w363:errorcluster)  [unwired: 3 out]
      n489 = Release Queue(queue=w349, error in (no error)=w348) -> (error out=w347:errorcluster)  [unwired: 3 out]
      n490 = Release Queue(queue=w346, error in (no error)=w345) -> (error out=w344:errorcluster)  [unwired: 3 out]
      n491 = call <vilib>:"Simple Error Handler.vi"("error in (no error)"=w363) -> ()  [unwired: 1 in, 8 out]
      n492 = call <vilib>:"Simple Error Handler.vi"("error in (no error)"=w290) -> ()  [unwired: 1 in, 8 out]
      n493 = call <vilib>:"Simple Error Handler.vi"("error in (no error)"=w347) -> ()  [unwired: 1 in, 8 out]
      n494 = call <vilib>:"Simple Error Handler.vi"("error in (no error)"=w344) -> ()  [unwired: 1 in, 8 out]
      n495 = call <vilib>:"Simple Error Handler.vi"("error in (no error)"=w354) -> ()  [unwired: 4 in, 5 out]
      n496 = Release Queue(queue=w365, error in (no error)=w366) -> (error out=w367:errorcluster)  [unwired: 3 out]
      n497 = call <vilib>:"Simple Error Handler.vi"("error in (no error)"=w367) -> ()  [unwired: 1 in, 8 out]
      n498 = while {
        tunnel: [w557] -> w343
        tunnel: w272 -> [w553]
        tunnel: w273 -> [w554]
        tunnel: w258 -> [w542]
        tunnel: w262 -> [w544]
        tunnel: [w543] -> w341
        tunnel: w259 -> [w541]
        shift-right: [w539] -> _
        shift-left: w265 -> [w540]
        stop <- w545 stop-if-true
        # "[MIL] WORKER VI\nExecute upon 'mainq' commands\n - operates on slave timebase"
        n499 = Get Queue Status(queue=w554, error in (no error)=w553) -> (queue out=w543:refnum<queue>, error out=w557:errorcluster)  [unwired: 7 out]
        n500 = Dequeue Element(queue=w554, error in (no error)=w553) -> (queue out=w549:refnum<queue>, element=w548:cluster{string, string, variant}, error out=w556:errorcluster)  [unwired: 1 in, 1 out]
        n501 = Unbundle(w548) -> (w555:string, w551:string, w550:variant)
        n502 = case shown="\"MIL\"" w551 {
          tunnel: w556 -> [w563 w570 w574]
          tunnel: w555 -> [w561 w568 _]
          tunnel: [w562 w569 ""] -> w552
          tunnel: w550 -> [w559 w566 _]
          tunnel: w549 -> [_ _ w576]
          tunnel: w548 -> [_ _ w575]
          tunnel: w542 -> [w560 w567 _]
          tunnel: w541 -> [_ _ _]
          tunnel: w540 -> [w558 w565 w572]
          tunnel: [w558 w565 w572] -> w539
          frame "MIL" {
            n503 = case shown="Default" w561 {
              tunnel: w563 -> [_]
              tunnel: [""] -> w562
              tunnel: w560 -> [_]
              tunnel: w559 -> [_]
              frame Default {
              }
            }
          }
          frame "placeholder" {
            n504 = case shown="Default" w568 {
              tunnel: w570 -> [_]
              tunnel: [""] -> w569
              tunnel: w567 -> [_]
              tunnel: w566 -> [_]
              frame Default {
              }
            }
          }
          frame Default {
            n505 = Enqueue Element(queue=w576, element=w575, error in (no error)=w574) -> ()  [unwired: 1 in, 3 out]
          }
        }
        n506 = Unbundle By Name(w557) -> ("status"=w545:bool)
        n507 = Scale By Power Of 2(n=0, x=w544) -> (x*2^n=w546:dbl)
        n508 = Wait Until Next ms Multiple(millisecond multiple=w546) -> ()  [unwired: 1 out]
        n509 = call "writeNotification.vi"("string"=w552, "Array"=w542) -> ()  [unwired: 10 in]
      }
      n510 = while {
        tunnel: [w526] -> w340
        tunnel: w270 -> [w522]
        tunnel: w271 -> [w523]
        tunnel: w258 -> [w511]
        tunnel: w262 -> [w513]
        tunnel: [w512] -> w338
        tunnel: w259 -> [w510]
        shift-right: [w508] -> _
        shift-left: w265 -> [w509]
        stop <- w514 stop-if-true
        # "[unused] WORKER VII\nExecute upon 'mainq' commands\n - operates on slave timebase"
        n511 = Get Queue Status(queue=w523, error in (no error)=w522) -> (queue out=w512:refnum<queue>, error out=w526:errorcluster)  [unwired: 7 out]
        n512 = Dequeue Element(queue=w523, error in (no error)=w522) -> (queue out=w518:refnum<queue>, element=w517:cluster{string, string, variant}, error out=w525:errorcluster)  [unwired: 1 in, 1 out]
        n513 = Unbundle(w517) -> (w524:string, w520:string, w519:variant)
        n514 = case shown="\"placeholder\"" w520 {
          tunnel: w525 -> [w532 w536]
          tunnel: w524 -> [w530 _]
          tunnel: [w531 ""] -> w521
          tunnel: w519 -> [w528 _]
          tunnel: w518 -> [_ w538]
          tunnel: w517 -> [_ w537]
          tunnel: w511 -> [w529 _]
          tunnel: w510 -> [_ _]
          tunnel: w509 -> [w527 w534]
          tunnel: [w527 w534] -> w508
          frame "placeholder" {
            n515 = case shown="Default" w530 {
              tunnel: w532 -> [_]
              tunnel: [""] -> w531
              tunnel: w529 -> [_]
              tunnel: w528 -> [_]
              frame Default {
              }
            }
          }
          frame Default {
            n516 = Enqueue Element(queue=w538, element=w537, error in (no error)=w536) -> ()  [unwired: 1 in, 3 out]
          }
        }
        n517 = Unbundle By Name(w526) -> ("status"=w514:bool)
        n518 = Scale By Power Of 2(n=0, x=w513) -> (x*2^n=w515:dbl)
        n519 = Wait Until Next ms Multiple(millisecond multiple=w515) -> ()  [unwired: 1 out]
        n520 = call "writeNotification.vi"("string"=w521, "Array"=w511) -> ()  [unwired: 10 in]
      }
      n521 = while {
        tunnel: [w495] -> w337
        tunnel: w268 -> [w491]
        tunnel: w269 -> [w492]
        tunnel: w258 -> [w480]
        tunnel: w262 -> [w482]
        tunnel: [w481] -> w335
        tunnel: w259 -> [w479]
        shift-right: [w477] -> _
        shift-left: w265 -> [w478]
        stop <- w483 stop-if-true
        # "[unused] WORKER VIII\nExecute upon 'mainq' commands\n - operates on slave timebase"
        n522 = Get Queue Status(queue=w492, error in (no error)=w491) -> (queue out=w481:refnum<queue>, error out=w495:errorcluster)  [unwired: 7 out]
        n523 = Dequeue Element(queue=w492, error in (no error)=w491) -> (queue out=w487:refnum<queue>, element=w486:cluster{string, string, variant}, error out=w494:errorcluster)  [unwired: 1 in, 1 out]
        n524 = Unbundle(w486) -> (w493:string, w489:string, w488:variant)
        n525 = case shown="Default" w489 {
          tunnel: w494 -> [w501 w505]
          tunnel: w493 -> [w499 _]
          tunnel: [w500 ""] -> w490
          tunnel: w488 -> [w497 _]
          tunnel: w487 -> [_ w507]
          tunnel: w486 -> [_ w506]
          tunnel: w480 -> [w498 _]
          tunnel: w479 -> [_ _]
          tunnel: w478 -> [w496 w503]
          tunnel: [w496 w503] -> w477
          frame "placeholder" {
            n526 = case shown="Default" w499 {
              tunnel: w501 -> [_]
              tunnel: [""] -> w500
              tunnel: w498 -> [_]
              tunnel: w497 -> [_]
              frame Default {
              }
            }
          }
          frame Default {
            n527 = Enqueue Element(queue=w507, element=w506, error in (no error)=w505) -> ()  [unwired: 1 in, 3 out]
          }
        }
        n528 = Unbundle By Name(w495) -> ("status"=w483:bool)
        n529 = Scale By Power Of 2(n=0, x=w482) -> (x*2^n=w484:dbl)
        n530 = Wait Until Next ms Multiple(millisecond multiple=w484) -> ()  [unwired: 1 out]
        n531 = call "writeNotification.vi"("string"=w490, "Array"=w480) -> ()  [unwired: 10 in]
      }
      n532 = while {
        tunnel: [w464] -> w294
        tunnel: w266 -> [w460]
        tunnel: w267 -> [w461]
        tunnel: w258 -> [w449]
        tunnel: w262 -> [w451]
        tunnel: [w450] -> w292
        tunnel: w259 -> [w448]
        shift-right: [w446] -> _
        shift-left: w265 -> [w447]
        stop <- w452 stop-if-true
        # "[unused] WORKER IX\nExecute upon 'mainq' commands\n - operates on slave timebase"
        n533 = Get Queue Status(queue=w461, error in (no error)=w460) -> (queue out=w450:refnum<queue>, error out=w464:errorcluster)  [unwired: 7 out]
        n534 = Dequeue Element(queue=w461, error in (no error)=w460) -> (queue out=w456:refnum<queue>, element=w455:cluster{string, string, variant}, error out=w463:errorcluster)  [unwired: 1 in, 1 out]
        n535 = Unbundle(w455) -> (w462:string, w458:string, w457:variant)
        n536 = case shown="Default" w458 {
          tunnel: w463 -> [w470 w474]
          tunnel: w462 -> [w468 _]
          tunnel: [w469 ""] -> w459
          tunnel: w457 -> [w466 _]
          tunnel: w456 -> [_ w476]
          tunnel: w455 -> [_ w475]
          tunnel: w449 -> [w467 _]
          tunnel: w448 -> [_ _]
          tunnel: w447 -> [w465 w472]
          tunnel: [w465 w472] -> w446
          frame "placeholder" {
            n537 = case shown="Default" w468 {
              tunnel: w470 -> [_]
              tunnel: [""] -> w469
              tunnel: w467 -> [_]
              tunnel: w466 -> [_]
              frame Default {
              }
            }
          }
          frame Default {
            n538 = Enqueue Element(queue=w476, element=w475, error in (no error)=w474) -> ()  [unwired: 1 in, 3 out]
          }
        }
        n539 = Unbundle By Name(w464) -> ("status"=w452:bool)
        n540 = Scale By Power Of 2(n=0, x=w451) -> (x*2^n=w453:dbl)
        n541 = Wait Until Next ms Multiple(millisecond multiple=w453) -> ()  [unwired: 1 out]
        n542 = call "writeNotification.vi"("string"=w459, "Array"=w449) -> ()  [unwired: 10 in]
      }
      n543 = Release Queue(queue=w341, error in (no error)=w343) -> (error out=w342:errorcluster)  [unwired: 3 out]
      n544 = Release Queue(queue=w338, error in (no error)=w340) -> (error out=w339:errorcluster)  [unwired: 3 out]
      n545 = Release Queue(queue=w292, error in (no error)=w294) -> (error out=w293:errorcluster)  [unwired: 3 out]
      n546 = Release Queue(queue=w335, error in (no error)=w337) -> (error out=w336:errorcluster)  [unwired: 3 out]
      n547 = call <vilib>:"Simple Error Handler.vi"("error in (no error)"=w342) -> ()  [unwired: 1 in, 8 out]
      n548 = call <vilib>:"Simple Error Handler.vi"("error in (no error)"=w339) -> ()  [unwired: 1 in, 8 out]
      n549 = call <vilib>:"Simple Error Handler.vi"("error in (no error)"=w336) -> ()  [unwired: 1 in, 8 out]
      n550 = call <vilib>:"Simple Error Handler.vi"("error in (no error)"=w293) -> ()  [unwired: 1 in, 8 out]
      n551 = call-poly <vilib>:"Create Timing Source.vi"("name (in)"="BlinkTimer1") -> ("name (out)"=w257:string)  [unwired: 9 in, 1 out]
      n552 = node-c288(w257, w255, "LIAconn_blink") -> (w261:T6)  [unwired: 7 in]
      n553 = timed-loop {
        timing: w261 -> [_]
        timing-out: [_] -> w260
        tunnel: w259 -> [w375]
        tunnel: w258 -> [w368]
        tunnel: w255 -> [w369]
        i -> [w374]
        stop <- w372 stop-if-true
        n554 = node-c288() -> (w373:errorcluster)  [unwired: 1 in]
        n555 = local read "LIAtimer1"() -> (w371:bool)
        n556 = case shown="False" w371 {
          tunnel: w375 -> [_ w390]
          tunnel: w374 -> [_ w387]
          tunnel: [w377 w381] -> w372
          tunnel: w373 -> [w377 w382]
          tunnel: [w376 w378] -> w370
          tunnel: w369 -> [w376 w380]
          tunnel: w368 -> [_ w379]
          frame False {
          }
          frame True {
            n557 = Quotient & Remainder(x=w387, y=2) -> (x-y*floor(x/y)=w386:i32)  [unwired: 1 out]
            n558 = Equal To 0?(x=w386) -> (x = 0?=w384:bool)
            n559 = Unbundle(w390) -> (w391:cluster{string, "qintoMain":refnum<user-event>})  [unwired: 1 out]
            n560 = And(x=w384, y=TRUE) -> (x .and. y?=w385:bool)
            n561 = call "findBlinkTimeLIA.vi"("refarr"=w379, "maxperiod"=w380) -> ("adjustedperiod"=w378:i32)
            n562 = To Variant(anything=w385) -> (Variant=w389:variant)
            n563 = Bundle("LIAconn", "updui", "Variant"=w389) -> (w392:cluster{string, string, "Variant":variant})  [unwired: 1 in]
            n564 = Build Array(w392) -> (w393:cluster{string, string, "Variant":variant}[])
            n565 = call "enqMulti.vi"("error in (no error)"=w382, "array of cmds"=w393, "eventcluster"=w391) -> ("error out"=w381:errorcluster)  [unwired: 8 in]
          }
        }
        n566 = node-c288(w372, w370) -> ()  [unwired: 6 in, 1 out]
      }
      n567 = node-c288(w260) -> ()
    }
  }
